vi "运维调试_总磷总氮.vi"() -> ()   [LabVIEW 2016, in "斯坦道总磷.lvlib"]
uses:
  <vilib>/Utility/miscctls.llb/LVStringsAndValuesArrayTypeDef_U16.ctl
  <vilib>/Utility/miscctls.llb/LVPointTypeDef.ctl
  <vilib>/Plasmionique/MB Master/MB_Master/MB_Master.lvclass
  <vilib>/Utility/config.llb/NI_LVConfig.lvlib
  <vilib>/ptbypt/NI_PtbyPt.lvlib
panel:
  in  "灯值调整":bool
  in  "测试量程配置":T1
  in  "启动参数设置":bool
  out "固件版本号":string
  in  "定时设置":cluster{"启动":bool, "控制命令":T2, "测量参数":T3}(xcontrol)
  out "模块版本号":string
  out "温度2":sgl
  out "温度1":sgl
  out "ADC":sgl
  out "F3":sgl format="%#.6f"
  out "F2":sgl format="%#.6f"
  out "F1":sgl format="%#.6f"
  out "F0":sgl format="%#.6f"
  out "运行状态":T4 {"数据时间:" format="%<%y/%m/%d %H:%M:%S>T"; "仪器时间:" format="%<%y/%m/%d %H:%M:%S>T"}
  in  "单选按钮":enum32{"COD", "NH3N", "TN", "TP"}(radio)=enum."TN"
  in  "仪器参数":bool
  out "二级权限":bool
  out "一级权限":bool
  out "输入密码":u32
  out "布尔":bool
  in  "流程固件":bool
  in  "量程参数读取":T5
  in  "模块启用":bool
  in  "串口设置":bool
  in  "公式一键写入":bool
  in  "流程路径":path=path "data/流程.xml"
  in  "曲线模型":cluster{"X^2":dbl, "X":dbl, "B":dbl, "r^2":dbl}(xcontrol)
  out "字符串 2":string
  in  "质控参数设置":bool
  in  "数组":string[](array[string])
  in  "量程切换阈值写入":bool
  in  "量程切换阈值读取":bool
  in  "参数下拉列表":enum16{"COD", "氨氮", "总氮", "总磷"}(ring)
  in  "量程下拉列表":enum16{"低量程", "高量程"}(ring)
  in  "测量模式下拉列表":enum16{"水样测量", "零点核查", "跨度核查", "标样核查", "加标回收"}(ring)
  in  "公式":cluster{"X^2":dbl, "X":dbl, "b":dbl}
  in  "写公式":bool
  in  "读公式":bool
  in  "返回":bool
  in  "参数设置":bool
  out "集成报警信息":string
  in  "停止":bool
  in  "手动启动":bool
  in  "单步测试":bool
  out "多列列表框":i32(listbox)
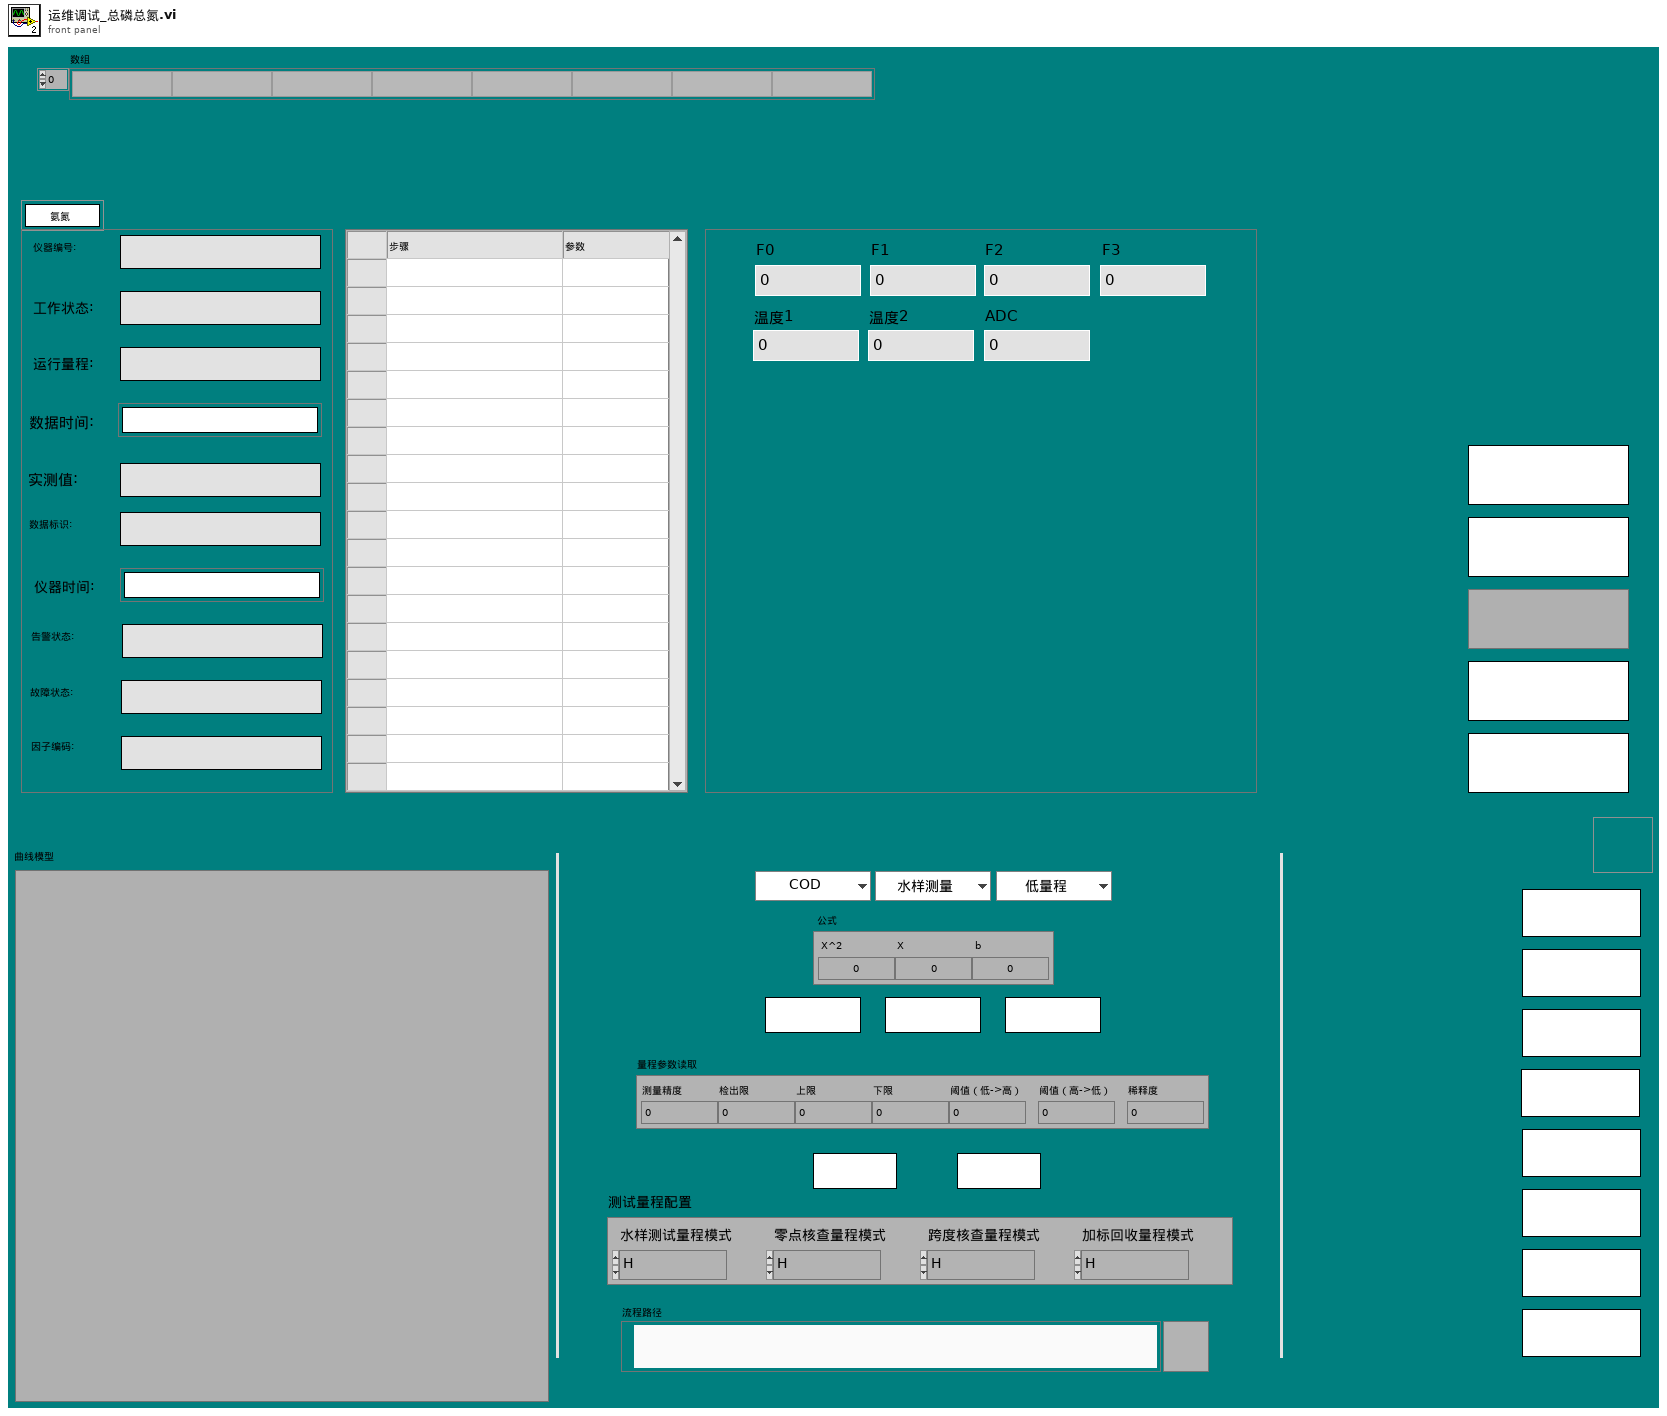
[diagram p1: front panel]
types:
  T1 = cluster{"水样测试量程模式":enum16{"H", "L", "AUTO"}, "空白核查量程模式":enum16{"H", "L", "AUTO"}, "跨度核查量程模式":enum16{"H", "L", "AUTO"}, "跨度核查量程模式 2":enum16{"H", "L", "AUTO"}}
  T2 = typedef "定时设置.xctl/国标控制命令.ctl" = enum16{"启动测量", "标样核查", "零点核查", "跨度核查", "空白测试", "平行样测试", "加标回收", "空白校准", "标样校准", "初始化（清洗）", "停止测试", "仪器重启", "校时", "模式设置", "测量间隔设置"}
  T3 = typedef "定时设置.xctl/测量参数.ctl" = u16
  T4 = cluster{"仪器编号:":string, "工作状态:":string, "运行量程: ":string, "数据时间:":timestamp, "实测值:":string, "数据标识: ":string, "仪器时间:":timestamp, "告警状态: ":string, "故障状态:  ":string, "因子编码:":string}
  T5 = cluster{"测量精度":dbl, "检出限":dbl, "上限":dbl, "下限":dbl, "阈值（低->高）":dbl, "阈值（高->低）":dbl, "稀释度":dbl}
  T6 = cluster{"时间源选择":enum16{"系统时间源", "仪器时间源"}, "外部时间源":timestamp}
  T7 = cluster{"系统时间":timestamp, "工作状态":enum16{"空闲", "水样测试", "标样核查", "零点核查", "跨度核查", "空白测试", "平行样测试", "加标回收", "空白校准", "标样校准", "初始化（清洗）"}, "测量模式":enum16{"待机", "连续模式", "周期模式", "定点模式", "受控模式", "手动模式"}, "告警代码":u16, "故障代码":u16, "日志代码":u16, "软件版本":u16, "F0":sgl, "F1":sgl, "F2":sgl, "F3":sgl, "T":sgl, "H":sgl, "id":u16, "flowid":u16, "量程":u16, "总磷控温温度1":sgl, "营养盐控温温度2":sgl, "ADC":sgl}
  T8 = enum32{"Bad", "Idle", "Run top level", "Running"}
  T9 = enum16{"空闲", "水样测试", "标样核查", "零点核查", "跨度核查", "空白测试", "平行样测试", "加标回收", "空白校准", "标样校准", "初始化（清洗）"}
  T10 = cluster{"水样测试量程模式":enum16{"H", "L", "AUTO"}, "空白核查量程模式":enum16{"H", "L", "AUTO"}, "跨度核查量程模式":enum16{"H", "L", "AUTO"}, "加标回收量程模式":enum16{"H", "L", "AUTO"}}
  T11 = typedef "LVStringsAndValuesArrayTypeDef_U16.ctl" = cluster{"String":string, "Value":u16}[]
  T12 = cluster{"COD":bool, "氨氮":bool, "总氮":bool, "总磷":bool}
  T13 = cluster{"参数下拉列表":enum16{"COD", "氨氮", "总氮", "总磷"}, "测量模式下拉列表":enum16{"水样测量", "零点核查", "跨度核查", "标样核查", "加标回收"}, "量程下拉列表":enum16{"低量程", "高量程"}}
  T14 = typedef "NI_LVConfig.lvlib/Config Data RefNum.ctl" = refnum<k1>
  T15 = cluster{"Major":u16, "Minor":u16, "Fix":u16, "Build":u16}
  T16 = typedef "LVPointTypeDef.ctl" = cluster{"Horizontal":i16, "Vertical":i16}
  T17 = cluster{"因子编码":u32, "单位":u16, "标样参考值":sgl, "水样数据时间":timestamp, "水样实测值":sgl, "水样数据标识":string, "标样数据时间":timestamp, "标样实测值":sgl, "标样数据标识":string, "空白数据时间":timestamp, "空白实测值":sgl, "空白数据标识":string, "零点核查数据时间":timestamp, "零点核查实测值":sgl, "零点核查数据标识":string, "跨度核查数据时间":timestamp, "跨度核查实测值":sgl, "跨度核查数据标识":string, "加标回收数据时间":timestamp, "加标回收实测值":sgl, "加标回收数据标识":string, "平行样数据时间":timestamp, "平行样实测值":sgl, "平行样数据标识":string, "F0":sgl, "F1":sgl, "F2":sgl, "F3":sgl, "F4":sgl, "F5":sgl, "F6":sgl, "F7":sgl, "温度":sgl, "湿度":sgl, "X值":sgl, "fidrange":u16}
  T18 = cluster{"时间标识":timestamp, "设备":string, "日志信息":string, "备注":string}
  T19 = cluster{"参数":string, "报警内容":string, "报警分析":string}
  T20 = cluster{"启动模式":enum16{"跨度核查", "水样测量", "空白核查", "标样核查", "加标回收"}, "启动参数":u16, "量程":enum16{"低量程", "高量程"}}
  T21 = cluster{"时间标识":timestamp, "设备":string, "日志信息":string, "流程参数":string}
  T22 = typedef "LVRowAndColumnUnsignedTypeDef.ctl" = cluster{"Row":u32, "Column":u32}
  T23 = cluster{"站号":u16, "量程切换":enum32{"H", "L", "AUTO"}, "控制命令":enum16{"启动测量", "标样核查", "零点核查", "跨度核查", "空白测试", "平行样测试", "加标回收", "空白校准", "标样校准", "初始化（清洗）", "停止测试", "仪器重启", "校时", "模式设置", "测量间隔设置"}, "模式设置":enum16{"待机", "连续模式", "周期模式", "定点模式", "受控模式", "手动模式"}, "测量间隔":u16}
  T24 = cluster{"被复制模型":cluster{"参数":u8, "测量模式":u8, "量程":u8}, "被覆盖模型":cluster{"参数":u8, "测量模式":u8, "量程":u8}[]}
  T25 = cluster{"总磷跨度值":dbl, "总磷零点标准液浓度":dbl, "总磷跨度标准液浓度":dbl, "总磷标准液标准浓度":dbl, "总氮跨度值":dbl, "总氮零点标准液浓度":dbl, "总氮跨度标准液浓度":dbl, "总氮标准液标准浓度":dbl, "COD跨度值":dbl, "COD零点标准液浓度":dbl, "COD跨度标准液浓度":dbl, "COD标准液标准浓度":dbl, "氨氮跨度值":dbl, "氨氮零点标准液浓度":dbl, "氨氮跨度标准液浓度":dbl, "氨氮标准液标准浓度":dbl}
  T26 = cluster{"测量量程":dbl, "测量精度":dbl, "测量间隔":dbl, "消解温度":dbl, "消解时长":dbl, "空白校准时间":timestamp, "曲线截距":dbl, "曲线斜率":dbl, "测量检出限":dbl, "测量信号值":dbl, "线性相关系数":dbl, "二次多项式系数":dbl, "标样校准时间":timestamp, "稀释倍数":dbl, "三项式系数":dbl, "空白标定系数":dbl, "量程系数":dbl, "F0/ORPA":dbl, "F1/ORPB":dbl, "F2/ORPK":dbl, "F3":dbl, "F4":dbl, "F5":dbl, "F6":dbl, "F7":dbl, "X0/滴定数":dbl, "量程":dbl}
  T27 = cluster{"COD仪器参数":cluster{"测量量程":dbl, "测量精度":dbl, "测量间隔":dbl, "消解温度":dbl, "消解时长":dbl, "空白校准时间":timestamp, "曲线截距":dbl, "曲线斜率":dbl, "测量检出限":dbl, "测量信号值":dbl, "线性相关系数":dbl, "二次多项式系数":dbl, "标样校准时间":timestamp, "稀释倍数":dbl, "三项式系数":dbl, "空白标定系数":dbl, "量程系数":dbl, "F0/ORPA":dbl, "F1/ORPB":dbl, "F2/ORPK":dbl, "F3":dbl, "F4":dbl, "F5":dbl, "F6":dbl, "F7":dbl, "X0/滴定数":dbl, "量程":dbl}, "氨氮仪器参数":cluster{"测量量程":dbl, "测量精度":dbl, "测量间隔":dbl, "消解温度":dbl, "消解时长":dbl, "空白校准时间":timestamp, "曲线截距":dbl, "曲线斜率":dbl, "测量检出限":dbl, "测量信号值":dbl, "线性相关系数":dbl, "二次多项式系数":dbl, "标样校准时间":timestamp, "稀释倍数":dbl, "三项式系数":dbl, "空白标定系数":dbl, "量程系数":dbl, "F0/ORPA":dbl, "F1/ORPB":dbl, "F2/ORPK":dbl, "F3":dbl, "F4":dbl, "F5":dbl, "F6":dbl, "F7":dbl, "X0/滴定数":dbl, "量程":dbl}, "总氮仪器参数":cluster{"测量量程":dbl, "测量精度":dbl, "测量间隔":dbl, "消解温度":dbl, "消解时长":dbl, "空白校准时间":timestamp, "曲线截距":dbl, "曲线斜率":dbl, "测量检出限":dbl, "测量信号值":dbl, "线性相关系数":dbl, "二次多项式系数":dbl, "标样校准时间":timestamp, "稀释倍数":dbl, "三项式系数":dbl, "空白标定系数":dbl, "量程系数":dbl, "F0/ORPA":dbl, "F1/ORPB":dbl, "F2/ORPK":dbl, "F3":dbl, "F4":dbl, "F5":dbl, "F6":dbl, "F7":dbl, "X0/滴定数":dbl, "量程":dbl}, "总磷仪器参数":cluster{"测量量程":dbl, "测量精度":dbl, "测量间隔":dbl, "消解温度":dbl, "消解时长":dbl, "空白校准时间":timestamp, "曲线截距":dbl, "曲线斜率":dbl, "测量检出限":dbl, "测量信号值":dbl, "线性相关系数":dbl, "二次多项式系数":dbl, "标样校准时间":timestamp, "稀释倍数":dbl, "三项式系数":dbl, "空白标定系数":dbl, "量程系数":dbl, "F0/ORPA":dbl, "F1/ORPB":dbl, "F2/ORPK":dbl, "F3":dbl, "F4":dbl, "F5":dbl, "F6":dbl, "F7":dbl, "X0/滴定数":dbl, "量程":dbl}}
  T28 = cluster{"测量精度":u16, "检出限":dbl, "上限":dbl, "下限":dbl, "阈值（低->高）":dbl, "阈值（高->低）":dbl, "稀释度":dbl}
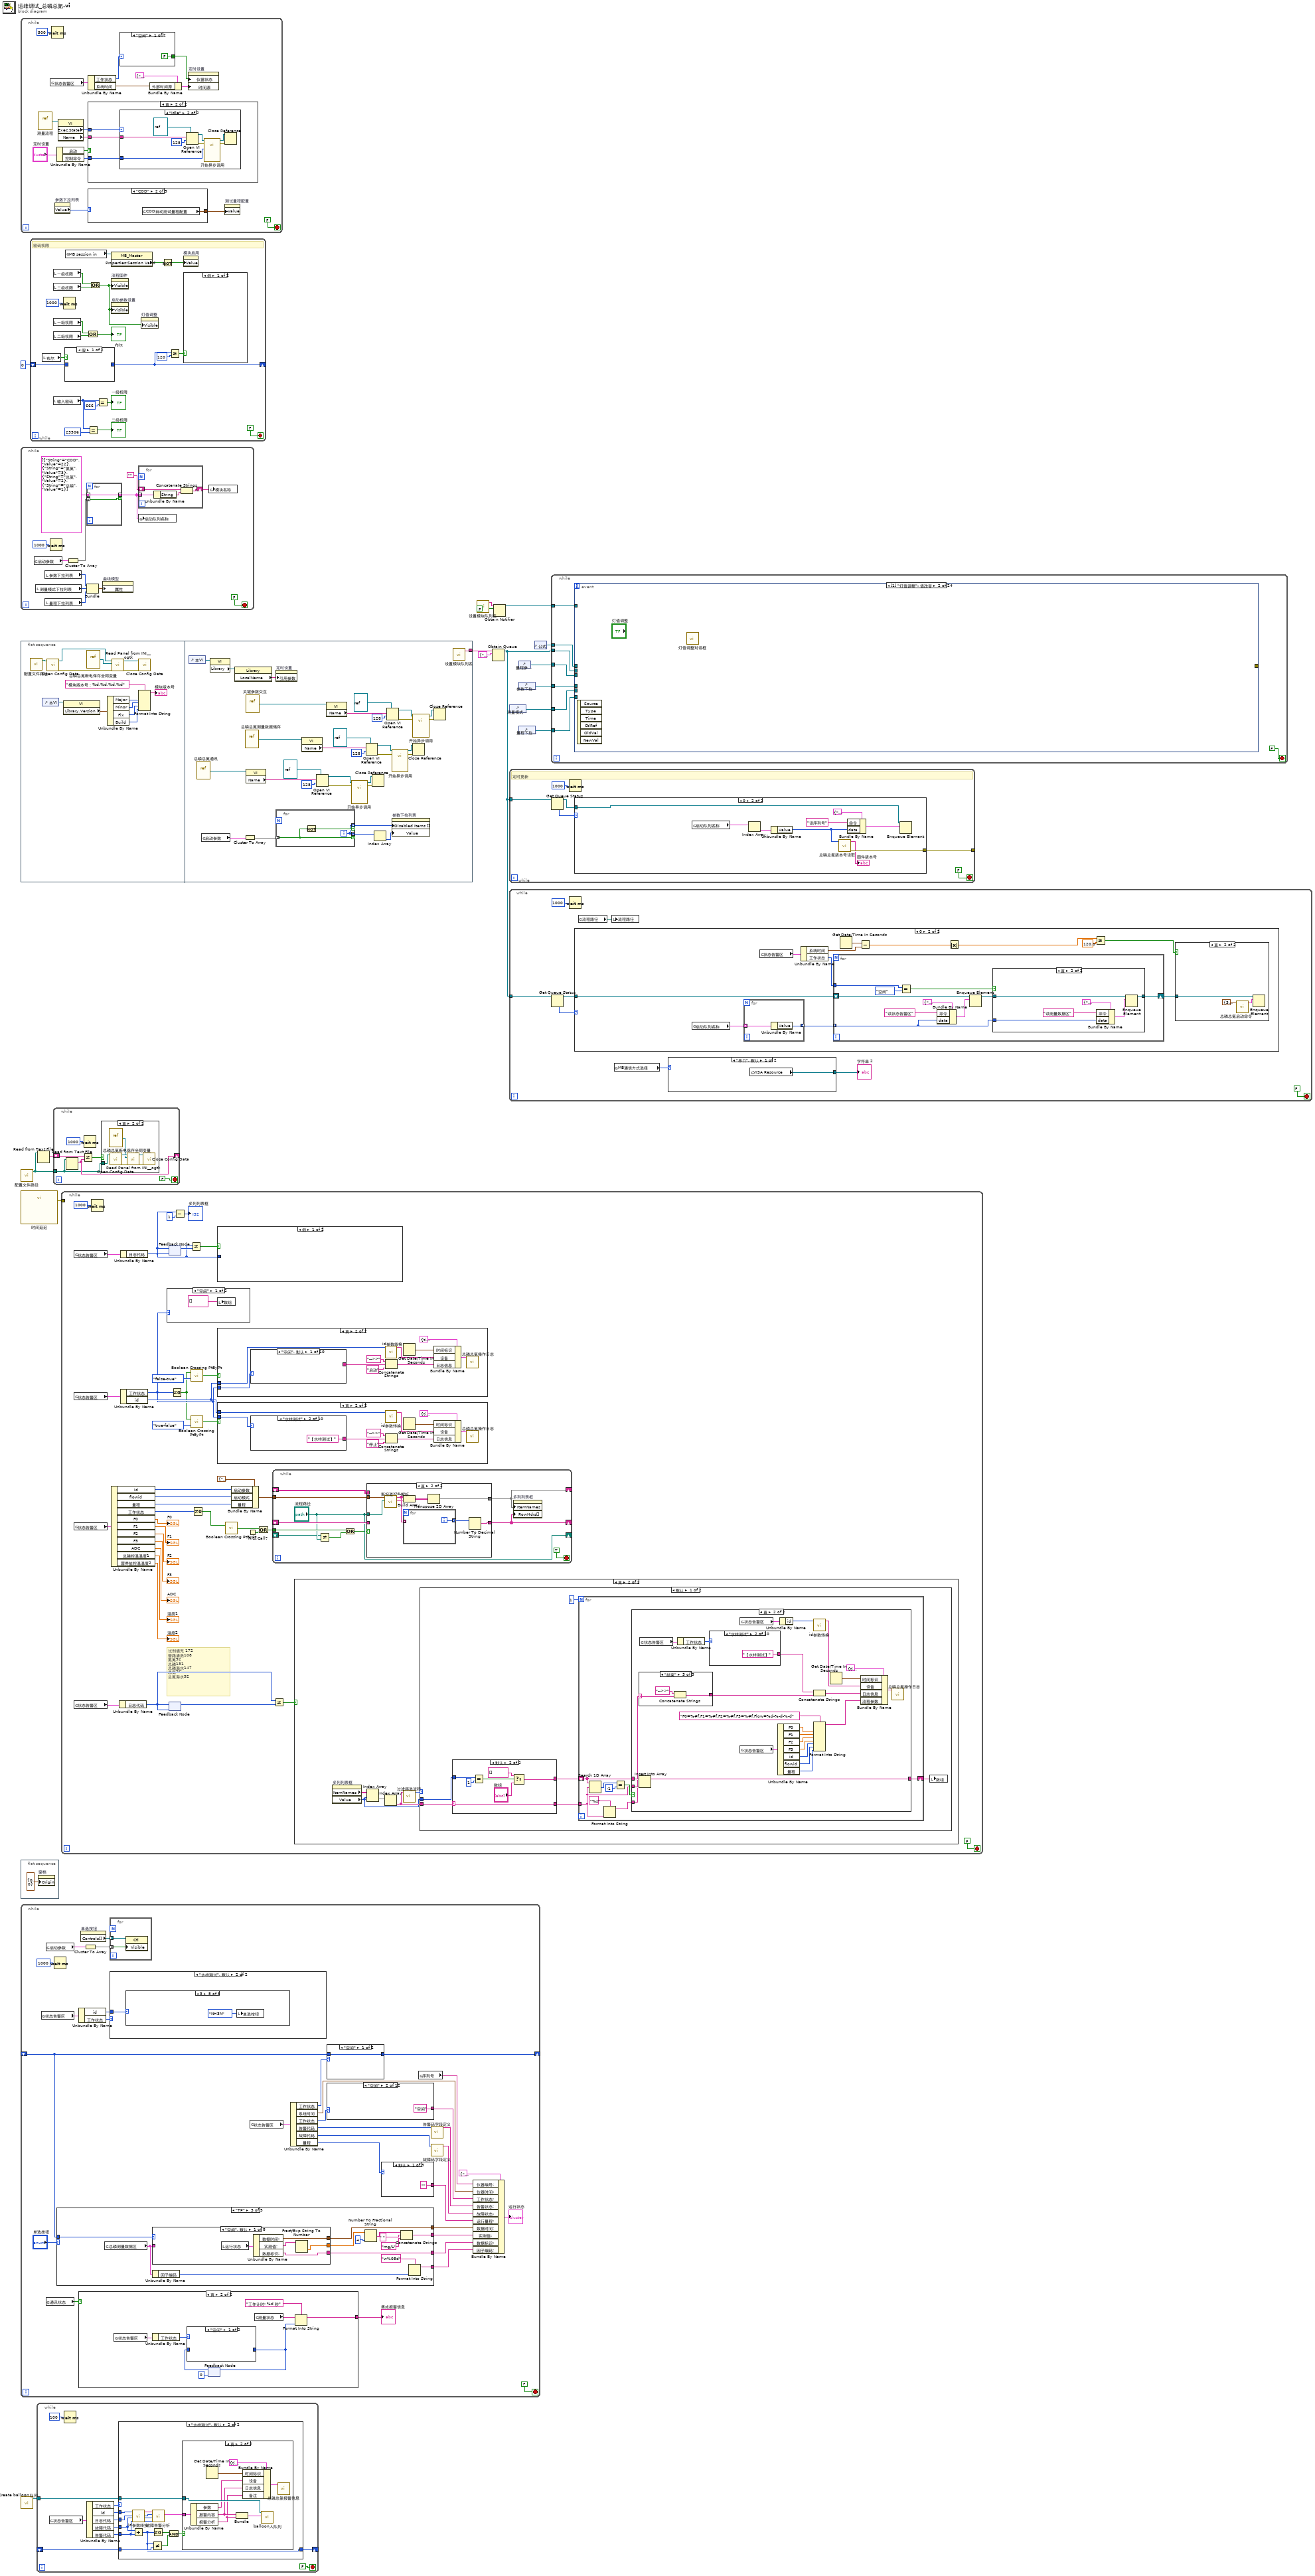
[diagram p0: block diagram]
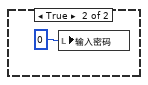
[diagram p5: hidden frame]
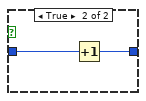
[diagram p6: hidden frame]
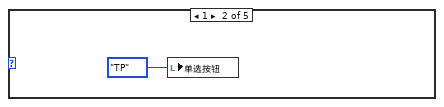
[diagram p11: hidden frame]
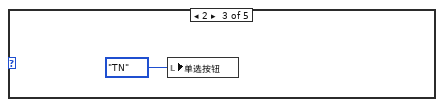
[diagram p12: hidden frame]
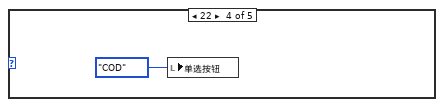
[diagram p13: hidden frame]
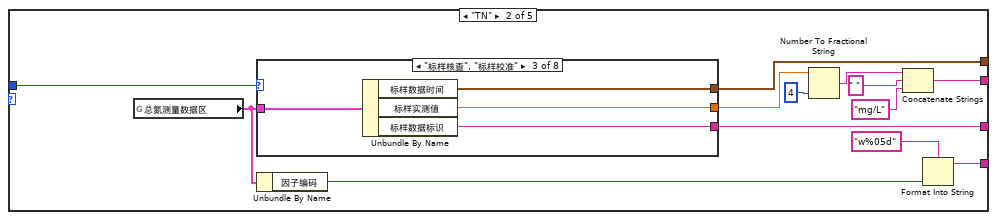
[diagram p15: hidden frame]
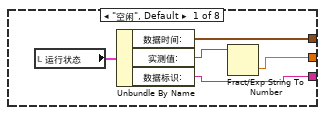
[diagram p16: hidden frame]
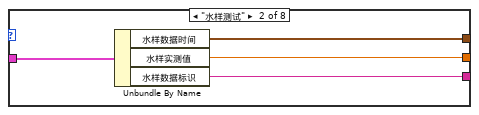
[diagram p17: hidden frame]
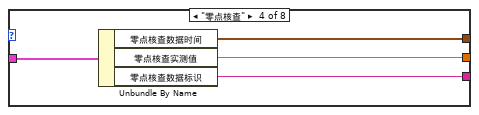
[diagram p18: hidden frame]
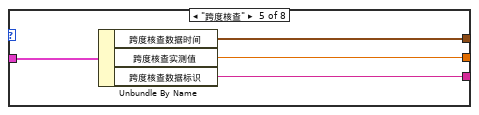
[diagram p19: hidden frame]
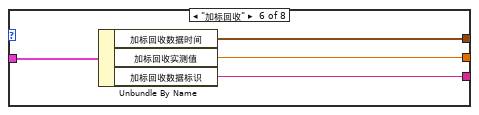
[diagram p20: hidden frame]
diagram:
  n1 = while {
    stop <- FALSE stop-if-true
    n2 = vi-ref "测量流程.vi"() -> (w30:refnum<vi>)
    n3 = global read "VAR总磷总氮全局变量.vi" "状态告警区"() -> (w27:T7)
    n4 = Wait (ms)(milliseconds to wait=u32 500 ("等待时间（毫秒）")) -> ()  [unwired: 1 out]
    n5 = property on="参数下拉列表" class="Enum (严格)"() -> ("Value"=w19:enum16{"COD", "氨氮", "总氮", "总磷"})  [unwired: 2 in, 2 out]
    n6 = Unbundle By Name("定时设置") -> ("启动"=w24:bool, "控制命令"=w23:T2)
    n7 = property class="VI"(reference=w30) -> ("Exec.State"=w29:T8, "Name"=w28:string)  [unwired: 1 in, 2 out]
    n8 = Unbundle By Name(w27) -> ("工作状态"=w26:T9, "系统时间"=w21:timestamp)
    n9 = case shown="真" w24 {
      tunnel: w28 -> [_ w41]
      tunnel: w23 -> [_ w40]
      tunnel: w29 -> [_ w39]
      frame False {
      }
      frame True {
        n10 = case shown="\"Idle\"" w39 {
          tunnel: w41 -> [_ w45]
          tunnel: w40 -> [_ w42]
          frame "Bad", Default {
          }
          frame "Idle" {
            n11 = Open VI Reference(type specifier VI Refnum (for type only)=refnum<vi> refnum, vi path=w45, options=128 ("选项")) -> (vi reference=w46:refnum<vi>, error out=w47:errorcluster)  [unwired: 3 in]
            n12 = call-by-ref "开始异步调用"(reference=w46, error in=w47, "控制命令"=w42) -> (reference out=w48:refnum<vi>, error out=w49:errorcluster)  [unwired: 11 in]
            n13 = Close Reference(reference=w48, error in (no error)=w49) -> ()  [unwired: 1 out]
          }
        }
      }
    }
    n14 = case shown="\"COD\"" w19 {
      tunnel: [_ w33 w34 w35 w36] -> w18
      frame Default {
      }
      frame "COD" {
        n15 = global read "总磷总氮断电保存全局变量.vi" "COD自动测试量程配置"() -> (w33:T10)
      }
      frame "氨氮" {
        n16 = global read "总磷总氮断电保存全局变量.vi" "氨氮自动测试量程配置"() -> (w34:T10)
      }
      frame "总氮" {
        n17 = global read "总磷总氮断电保存全局变量.vi" "总氮自动测试量程配置"() -> (w35:T10)
      }
      frame "总磷" {
        n18 = global read "总磷总氮断电保存全局变量.vi" "总磷自动测试量程配置"() -> (w36:T10)
      }
    }
    n19 = case shown="\"空闲\"" w26 {
      tunnel: [FALSE TRUE] -> w17
      frame "空闲" {
      }
      frame "水样测试", Default {
      }
    }
    n20 = Bundle By Name(cluster=T6 {"时间源选择"=enum."仪器时间源", "外部时间源"=timestamp(0 s since 1904-01-01)} ("时间源"), "外部时间源"=w21) -> (w20:T6)
    n21 = property on="定时设置" class="定时设置 (严格)"("仪器状态"=w17, "时间源"=w20) -> ()  [unwired: 2 in, 2 out]
    n22 = property on="测试量程配置" class="Clust (严格)"("Value"=w18) -> ()  [unwired: 2 in, 2 out]
  }
  n23 = while {
    stop <- FALSE stop-if-true
    n24 = global read "总磷总氮断电保存全局变量.vi" "启动参数"() -> (w59:T12)
    n25 = local read "测量模式下拉列表"() -> (w52:enum16{"水样测量", "零点核查", "跨度核查", "标样核查", "加标回收"})
    n26 = local read "参数下拉列表"() -> (w50:enum16{"COD", "氨氮", "总氮", "总磷"})
    n27 = local read "量程下拉列表"() -> (w51:enum16{"低量程", "高量程"})
    n28 = Wait (ms)(milliseconds to wait=u32 1000 ("等待时间（毫秒）")) -> ()  [unwired: 1 out]
    n29 = Cluster To Array(cluster=w59) -> (array=w58:bool[])
    n30 = for {
      tunnel: w58 -> [w67] mode=indexing
      tunnel: T11 [{"String"="COD", "Value"=22}, {"String"="氨氮", "Value"=3}, {"String"="总氮", "Value"=2}, {"String"="总磷", "Value"=1}] ("字符串与值[]") -> [w66] mode=indexing
      tunnel: [w66] -> w56 mode=indexing if=w67
    }
    n31 = Bundle("参数下拉列表"=w50, "测量模式下拉列表"=w52, "量程下拉列表"=w51) -> (w53:T13)  [unwired: 1 in]
    n32 = property on="曲线模型" class="曲线模型 (严格)"("属性"=w53) -> ()  [unwired: 2 in, 2 out]
    n33 = for {
      tunnel: w56 -> [w65] mode=indexing
      shift-right: [w64] -> w54
      shift-left: "" -> [w62]
      n34 = Unbundle By Name(w65) -> ("String"=w63:string)
      n35 = Concatenate Strings(w62, w63) -> (w64:string)
    }
    n36 = global write "VAR总磷总氮全局变量.vi" "启动队列名称"(w56) -> ()
    n37 = global write "VAR总磷总氮全局变量.vi" "模块名称"(w54) -> ()
  }
  n38 = flat-sequence {
    tunnel: [w83] -> w6
    frame #0 {
      n39 = call "配置文件路径.vi"() -> ("appended path"=w76:path)  [unwired: 11 in]
      n40 = control-ref of="本VI"() -> (w75:refnum<vi>)
      n41 = call <vilib>:"Open Config Data.vi"("configuration file path"=w76) -> ("error out"=w80:errorcluster, "refnum"=w77:T14)  [unwired: 8 in, 1 out]
      n42 = property class="VI"(reference=w75) -> ("Library.Version"=w74:T15)  [unwired: 1 in, 2 out]
      n43 = vi-ref "总磷总氮断电保存全局变量.vi"() -> (w78:refnum<vi>)
      n44 = Unbundle By Name(w74) -> ("Major"=w72:u16, "Minor"=w71:u16, "Fix"=w70:u16, "Build"=w69:u16)
      n45 = call <userlib>:"Read Panel from INI__ogtk.vi"("error in (no error)"=w80, "VI ref"=w78, "refnum"=w77) -> ("error out"=w81:errorcluster, "refnum out"=w79:T14)  [unwired: 7 in]
      n46 = call <vilib>:"Close Config Data.vi"("error in (no error)"=w81, "refnum"=w79) -> ()  [unwired: 8 in, 2 out]
      n47 = Format Into String(format string="模块版本号：%d.%d.%d.%d" ("格式字符串"), w72, w71, w70, w69) -> (resulting string=→"模块版本号":string)  [unwired: 2 in, 1 out]
    }
    frame #1 {
      n48 = control-ref of="本VI"() -> (w84:refnum<vi>)
      n49 = vi-ref "总磷总氮通讯.vi"() -> (w99:refnum<vi>)
      n50 = global read "总磷总氮断电保存全局变量.vi" "启动参数"() -> (w87:T12)
      n51 = property class="VI"(reference=w84) -> ("Library"=w85:refnum<vi>)  [unwired: 1 in, 2 out]
      n52 = property class="Library"(reference=w85) -> ("LocalName"=w86:string)  [unwired: 1 in, 2 out]
      n53 = Cluster To Array(cluster=w87) -> (array=w88:bool[])
      n54 = vi-ref "总磷总氮测量数据储存.vi"() -> (w107:refnum<vi>)
      n55 = vi-ref "关键参数交互.vi"() -> (w98:refnum<vi>)
      n56 = property class="VI"(reference=w99) -> ("Name"=w100:string)  [unwired: 1 in, 2 out]
      n57 = property on="定时设置" class="定时设置 (严格)"("引用参数"=w86) -> ()  [unwired: 2 in, 2 out]
      n58 = for {
        tunnel: w88 -> [w115] mode=indexing
        tunnel: [w116] -> w90 mode=indexing if=w117
        tunnel: [w116] -> w89 mode=indexing if=w115
        i -> [w116]
        n59 = Not(x=w115) -> (.not. x?=w117:bool)
      }
      n60 = property class="VI"(reference=w107) -> ("Name"=w114:string)  [unwired: 1 in, 2 out]
      n61 = Open VI Reference(type specifier VI Refnum (for type only)=refnum<vi> refnum, vi path=w100, options=128 ("选项")) -> (vi reference=w102:refnum<vi>, error out=w104:errorcluster)  [unwired: 3 in]
      n62 = property class="VI"(reference=w98) -> ("Name"=w92:string)  [unwired: 1 in, 2 out]
      n63 = call-by-ref "开始异步调用"(reference=w102, error in=w104) -> (reference out=w106:refnum<vi>, error out=w105:errorcluster)  [unwired: 12 in]
      n64 = Open VI Reference(type specifier VI Refnum (for type only)=refnum<vi> refnum, vi path=w114, options=128 ("选项")) -> (vi reference=w112:refnum<vi>, error out=w110:errorcluster)  [unwired: 3 in]
      n65 = Close Reference(reference=w106, error in (no error)=w105) -> ()  [unwired: 1 out]
      n66 = Index Array(array=w89) -> (element=w82:i32)  [unwired: 1 in]
      n67 = Open VI Reference(type specifier VI Refnum (for type only)=refnum<vi> refnum, vi path=w92, options=128 ("选项")) -> (vi reference=w94:refnum<vi>, error out=w95:errorcluster)  [unwired: 3 in]
      n68 = call-by-ref "开始异步调用"(reference=w112, error in=w110) -> (reference out=w108:refnum<vi>, error out=w109:errorcluster)  [unwired: 12 in]
      n69 = property on="参数下拉列表" class="Enum (严格)"("Disabled Items []"=w90, "Value"=w82) -> ()  [unwired: 2 in, 2 out]
      n70 = call-by-ref "开始异步调用"(reference=w94, error in=w95) -> (reference out=w97:refnum<vi>, error out=w96:errorcluster)  [unwired: 12 in]
      n71 = Close Reference(reference=w108, error in (no error)=w109) -> ()  [unwired: 1 out]
      n72 = Close Reference(reference=w97, error in (no error)=w96) -> ()  [unwired: 1 out]
      n73 = call "设置模块队列名.vi"() -> ("Msg"=w83:string)  [unwired: 5 in]
    }
  }
  n74 = call "配置文件路径.vi"() -> ("appended path"=w4:path)  [unwired: 11 in]
  n75 = call "时间延迟"() -> ("error out"=w11:errorcluster)  [unwired: 11 in]
  n76 = flat-sequence {
    frame #0 {
      n77 = property on="窗格" class="Pane"("Origin"=T16 {"Horizontal"=0, "Vertical"=0} ("原点")) -> ()  [unwired: 2 in, 2 out]
    }
  }
  n78 = while {
    shift-right: [w120] -> _
    shift-left: _ -> [w119]
    stop <- FALSE stop-if-true
    n79 = global read "VAR总磷总氮全局变量.vi" "状态告警区"() -> (w131:T7)
    n80 = global read "总磷总氮断电保存全局变量.vi" "启动参数"() -> (w123:T12)
    n81 = global read "VAR总磷总氮全局变量.vi" "通讯状态"() -> (w147:bool)
    n82 = Wait (ms)(milliseconds to wait=u32 1000 ("等待时间（毫秒）")) -> ()  [unwired: 1 out]
    n83 = case shown="\"TP\"" "单选按钮" {
      tunnel: w119 -> [_ w163 w209 w255 w301]
      tunnel: [_ w162 w208 w253 w299] -> w135
      tunnel: [_ w161 w211 w257 w303] -> w134
      tunnel: [_ w160 w206 w251 w297] -> w133
      tunnel: [_ w159 w210 w256 w302] -> w132
      frame Default {
      }
      frame "TN" {
        n84 = global read "VAR总磷总氮全局变量.vi" "总氮测量数据区"() -> (w164:T17)
        n85 = case shown="\"标样核查\", \"标样校准\"" w163 {
          tunnel: [w174 w180 w184 w188 w192 w196 w200 w204] -> w162
          tunnel: [w172 w179 w183 w187 w190 w195 w199 w203] -> w166
          tunnel: [w175 w178 w182 w186 w189 w194 w198 w202] -> w160
          tunnel: w164 -> [_ w177 w181 w185 w191 w193 w197 w201]
          frame "空闲", Default {
            n86 = local read "运行状态"() -> (w176:T4)
            n87 = Unbundle By Name(w176) -> ("数据时间:"=w174:timestamp, "实测值:"=w173:string, "数据标识:"=w175:string)
            n88 = Fract/Exp String To Number(string=w173) -> (number=w172:dbl)  [unwired: 3 in, 1 out]
          }
          frame "水样测试" {
            n89 = Unbundle By Name(w177) -> ("水样数据时间"=w180:timestamp, "水样实测值"=w179:sgl, "水样数据标识"=w178:string)
          }
          frame "标样核查", "标样校准" {
            n90 = Unbundle By Name(w181) -> ("标样数据时间"=w184:timestamp, "标样实测值"=w183:sgl, "标样数据标识"=w182:string)
          }
          frame "零点核查" {
            n91 = Unbundle By Name(w185) -> ("零点核查数据时间"=w188:timestamp, "零点核查实测值"=w187:sgl, "零点核查数据标识"=w186:string)
          }
          frame "跨度核查" {
            n92 = Unbundle By Name(w191) -> ("跨度核查数据时间"=w192:timestamp, "跨度核查实测值"=w190:sgl, "跨度核查数据标识"=w189:string)
          }
          frame "加标回收" {
            n93 = Unbundle By Name(w193) -> ("加标回收数据时间"=w196:timestamp, "加标回收实测值"=w195:sgl, "加标回收数据标识"=w194:string)
          }
          frame "空白测试", "空白校准" {
            n94 = Unbundle By Name(w197) -> ("空白数据时间"=w200:timestamp, "空白实测值"=w199:sgl, "空白数据标识"=w198:string)
          }
          frame "平行样测试" {
            n95 = Unbundle By Name(w201) -> ("平行样数据时间"=w204:timestamp, "平行样实测值"=w203:sgl, "平行样数据标识"=w202:string)
          }
        }
        n96 = Unbundle By Name(w164) -> ("因子编码"=w170:u32)
        n97 = Number To Fractional String(number=w166, precision (6)=i16 4 ("精度(6)")) -> (F-format string=w168:string)  [unwired: 2 in]
        n98 = Concatenate Strings(w168, " " ("字符串"), "mg/L" ("字符串")) -> (w161:string)
        n99 = Format Into String(format string="w%05d" ("格式字符串"), w170) -> (resulting string=w159:string)  [unwired: 2 in, 1 out]
      }
      frame "TP" {
        n100 = global read "VAR总磷总氮全局变量.vi" "总磷测量数据区"() -> (w205:T17)
        n101 = case shown="\"空闲\", 默认" w209 {
          tunnel: [w220 w226 w230 w234 w238 w242 w246 w250] -> w208
          tunnel: [w218 w225 w229 w233 w236 w241 w245 w249] -> w207
          tunnel: [w221 w224 w228 w232 w235 w240 w244 w248] -> w206
          tunnel: w205 -> [_ w223 w227 w231 w237 w239 w243 w247]
          frame "空闲", Default {
            n102 = local read "运行状态"() -> (w222:T4)
            n103 = Unbundle By Name(w222) -> ("数据时间:"=w220:timestamp, "实测值:"=w219:string, "数据标识:"=w221:string)
            n104 = Fract/Exp String To Number(string=w219) -> (number=w218:dbl)  [unwired: 3 in, 1 out]
          }
          frame "水样测试" {
            n105 = Unbundle By Name(w223) -> ("水样数据时间"=w226:timestamp, "水样实测值"=w225:sgl, "水样数据标识"=w224:string)
          }
          frame "标样核查" {
            n106 = Unbundle By Name(w227) -> ("标样数据时间"=w230:timestamp, "标样实测值"=w229:sgl, "标样数据标识"=w228:string)
          }
          frame "零点核查" {
            n107 = Unbundle By Name(w231) -> ("零点核查数据时间"=w234:timestamp, "零点核查实测值"=w233:sgl, "零点核查数据标识"=w232:string)
          }
          frame "跨度核查" {
            n108 = Unbundle By Name(w237) -> ("跨度核查数据时间"=w238:timestamp, "跨度核查实测值"=w236:sgl, "跨度核查数据标识"=w235:string)
          }
          frame "加标回收" {
            n109 = Unbundle By Name(w239) -> ("加标回收数据时间"=w242:timestamp, "加标回收实测值"=w241:sgl, "加标回收数据标识"=w240:string)
          }
          frame "空白测试" {
            n110 = Unbundle By Name(w243) -> ("空白数据时间"=w246:timestamp, "空白实测值"=w245:sgl, "空白数据标识"=w244:string)
          }
          frame "平行样测试" {
            n111 = Unbundle By Name(w247) -> ("平行样数据时间"=w250:timestamp, "平行样实测值"=w249:sgl, "平行样数据标识"=w248:string)
          }
        }
        n112 = Unbundle By Name(w205) -> ("因子编码"=w216:u32)
        n113 = Number To Fractional String(number=w207, precision (6)=i16 4 ("精度(6)")) -> (F-format string=w214:string)  [unwired: 2 in]
        n114 = Concatenate Strings(w214, " " ("字符串"), "mg/L" ("字符串")) -> (w211:string)
        n115 = Format Into String(format string="w%05d" ("格式字符串"), w216) -> (resulting string=w210:string)  [unwired: 2 in, 1 out]
      }
      frame "NH3N" {
        n116 = global read "VAR总磷总氮全局变量.vi" "氨氮测量数据区"() -> (w254:T17)
        n117 = case shown="\"空闲\", 默认" w255 {
          tunnel: [w266 w272 w276 w280 w284 w288 w292 w296] -> w253
          tunnel: [w264 w271 w275 w279 w282 w287 w291 w295] -> w252
          tunnel: [w267 w270 w274 w278 w281 w286 w290 w294] -> w251
          tunnel: w254 -> [_ w269 w273 w277 w283 w285 w289 w293]
          frame "空闲", Default {
            n118 = local read "运行状态"() -> (w268:T4)
            n119 = Unbundle By Name(w268) -> ("数据时间:"=w266:timestamp, "实测值:"=w265:string, "数据标识:"=w267:string)
            n120 = Fract/Exp String To Number(string=w265) -> (number=w264:dbl)  [unwired: 3 in, 1 out]
          }
          frame "水样测试" {
            n121 = Unbundle By Name(w269) -> ("水样数据时间"=w272:timestamp, "水样实测值"=w271:sgl, "水样数据标识"=w270:string)
          }
          frame "标样核查" {
            n122 = Unbundle By Name(w273) -> ("标样数据时间"=w276:timestamp, "标样实测值"=w275:sgl, "标样数据标识"=w274:string)
          }
          frame "零点核查" {
            n123 = Unbundle By Name(w277) -> ("零点核查数据时间"=w280:timestamp, "零点核查实测值"=w279:sgl, "零点核查数据标识"=w278:string)
          }
          frame "跨度核查" {
            n124 = Unbundle By Name(w283) -> ("跨度核查数据时间"=w284:timestamp, "跨度核查实测值"=w282:sgl, "跨度核查数据标识"=w281:string)
          }
          frame "加标回收" {
            n125 = Unbundle By Name(w285) -> ("加标回收数据时间"=w288:timestamp, "加标回收实测值"=w287:sgl, "加标回收数据标识"=w286:string)
          }
          frame "空白测试" {
            n126 = Unbundle By Name(w289) -> ("空白数据时间"=w292:timestamp, "空白实测值"=w291:sgl, "空白数据标识"=w290:string)
          }
          frame "平行样测试" {
            n127 = Unbundle By Name(w293) -> ("平行样数据时间"=w296:timestamp, "平行样实测值"=w295:sgl, "平行样数据标识"=w294:string)
          }
        }
        n128 = Unbundle By Name(w254) -> ("因子编码"=w262:u32)
        n129 = Number To Fractional String(number=w252, precision (6)=i16 4 ("精度(6)")) -> (F-format string=w260:string)  [unwired: 2 in]
        n130 = Concatenate Strings(w260, " " ("字符串"), "mg/L" ("字符串")) -> (w257:string)
        n131 = Format Into String(format string="w%05d" ("格式字符串"), w262) -> (resulting string=w256:string)  [unwired: 2 in, 1 out]
      }
      frame "COD" {
        n132 = global read "VAR总磷总氮全局变量.vi" "COD测量数据区"() -> (w300:T17)
        n133 = case shown="\"空闲\", 默认" w301 {
          tunnel: [w312 w318 w322 w326 w330 w334 w338 w342] -> w299
          tunnel: [w310 w317 w321 w325 w328 w333 w337 w341] -> w298
          tunnel: [w313 w316 w320 w324 w327 w332 w336 w340] -> w297
          tunnel: w300 -> [_ w315 w319 w323 w329 w331 w335 w339]
          frame "空闲", Default {
            n134 = local read "运行状态"() -> (w314:T4)
            n135 = Unbundle By Name(w314) -> ("数据时间:"=w312:timestamp, "实测值:"=w311:string, "数据标识:"=w313:string)
            n136 = Fract/Exp String To Number(string=w311) -> (number=w310:dbl)  [unwired: 3 in, 1 out]
          }
          frame "水样测试" {
            n137 = Unbundle By Name(w315) -> ("水样数据时间"=w318:timestamp, "水样实测值"=w317:sgl, "水样数据标识"=w316:string)
          }
          frame "标样核查" {
            n138 = Unbundle By Name(w319) -> ("标样数据时间"=w322:timestamp, "标样实测值"=w321:sgl, "标样数据标识"=w320:string)
          }
          frame "零点核查" {
            n139 = Unbundle By Name(w323) -> ("零点核查数据时间"=w326:timestamp, "零点核查实测值"=w325:sgl, "零点核查数据标识"=w324:string)
          }
          frame "跨度核查" {
            n140 = Unbundle By Name(w329) -> ("跨度核查数据时间"=w330:timestamp, "跨度核查实测值"=w328:sgl, "跨度核查数据标识"=w327:string)
          }
          frame "加标回收" {
            n141 = Unbundle By Name(w331) -> ("加标回收数据时间"=w334:timestamp, "加标回收实测值"=w333:sgl, "加标回收数据标识"=w332:string)
          }
          frame "空白测试" {
            n142 = Unbundle By Name(w335) -> ("空白数据时间"=w338:timestamp, "空白实测值"=w337:sgl, "空白数据标识"=w336:string)
          }
          frame "平行样测试" {
            n143 = Unbundle By Name(w339) -> ("平行样数据时间"=w342:timestamp, "平行样实测值"=w341:sgl, "平行样数据标识"=w340:string)
          }
        }
        n144 = Unbundle By Name(w300) -> ("因子编码"=w308:u32)
        n145 = Number To Fractional String(number=w298, precision (6)=i16 4 ("精度(6)")) -> (F-format string=w306:string)  [unwired: 2 in]
        n146 = Concatenate Strings(w306, " " ("字符串"), "mg/L" ("字符串")) -> (w303:string)
        n147 = Format Into String(format string="w%05d" ("格式字符串"), w308) -> (resulting string=w302:string)  [unwired: 2 in, 1 out]
      }
    }
    n148 = Unbundle By Name(w131) -> ("id"=w130:u16, "工作状态"=w125:T9)
    n149 = case shown="真" w147 {
      tunnel: ["通讯异常" ("集成报警信息") w363] -> w146
      frame False {
      }
      frame True {
        n150 = global read "VAR总磷总氮全局变量.vi" "状态告警区"() -> (w369:T7)
        n151 = Unbundle By Name(w369) -> ("工作状态"=w368:T9)
        n152 = feedback #1(0) -> (w366:i32)
        n153 = case shown="\"空闲\"" w368 {
          tunnel: w366 -> [_ w371]
          tunnel: [_ w370] -> w364
          frame "空闲" {
          }
          frame Default {
            n154 = Increment(x=w371) -> (x+1=w370:i32)
          }
        }
        n155 = feedback-in #1(w364) -> ()
        n156 = global read "VAR总磷总氮全局变量.vi" "测量状态"() -> (w362:string)
        n157 = Format Into String(format string="工作计时: %d 秒" ("格式字符串"), initial string=w362, w364) -> (resulting string=w363:string)  [unwired: 1 in, 1 out]
      }
    }
    "集成报警信息" <- w146
    n158 = property on="单选按钮" class="RadioBtnsControl (严格)"() -> ("Controls[]"=w124:refnum<vi>[])  [unwired: 2 in, 2 out]
    n159 = Cluster To Array(cluster=w123) -> (array=w122:bool[])
    n160 = for {
      tunnel: w124 -> [w153] mode=indexing
      tunnel: w122 -> [w152] mode=indexing
      n161 = property class="Ctl"(reference=w153, "Visible"=w152) -> ()  [unwired: 1 in, 2 out]
    }
    n162 = case shown="\"水样测试\", 默认" w125 {
      tunnel: w130 -> [_ w154]
      frame "空闲" {
      }
      frame "水样测试", Default {
        n163 = case shown="3" w154 {
          frame 0, Default {
          }
          frame 1 {
            n164 = local write "单选按钮"(enum32{"COD", "NH3N", "TN", "TP"}."TP" ("单选按钮")) -> ()
          }
          frame 2 {
            n165 = local write "单选按钮"(enum32{"COD", "NH3N", "TN", "TP"}."TN" ("单选按钮")) -> ()
          }
          frame 22 {
            n166 = local write "单选按钮"(enum32{"COD", "NH3N", "TN", "TP"}."COD" ("单选按钮")) -> ()
          }
          frame 3 {
            n167 = local write "单选按钮"(enum32{"COD", "NH3N", "TN", "TP"}."NH3N" ("单选按钮")) -> ()
          }
        }
      }
    }
    n168 = global read "VAR总磷总氮全局变量.vi" "状态告警区"() -> (w145:T7)
    n169 = Unbundle By Name(w145) -> ("工作状态"=w121:T9, "系统时间"=w141:timestamp, "工作状态"=w140:T9, "告警代码"=w129:u16, "故障代码"=w127:u16, "量程"=w138:u16)
    n170 = case shown="\"空闲\"" w121 {
      selector: w121 -> [_ w151]
      tunnel: [w150 w151] -> w120
      tunnel: w119 -> [w150 _]
      frame "空闲" {
      }
      frame "水样测试", Default {
      }
    }
    n171 = case shown="\"空闲\"" w140 {
      selector: w140 -> [w346 _ _ _ _ _ _ _ _ _ _ _]
      tunnel: [w347 "空闲" ("工作状态") "水样测量" ("工作状态") "标样核查" ("工作状态") "零点核查" ("工作状态") "跨度核查" ("工作状态") "空白测试" ("工作状态") "平行样测试" ("工作状态") "加标回收" ("工作状态") "空白校准" ("工作状态") "标样校准" ("工作状态") "初始化" ("工作状态")] -> w139
      frame Default {
        n172 = Format Into String(format string="%d" ("格式字符串"), initial string="未知" ("工作状态"), w346) -> (resulting string=w347:string)  [unwired: 1 in, 1 out]
      }
      frame "空闲" {
      }
      frame "水样测试" {
      }
      frame "标样核查" {
      }
      frame "零点核查" {
      }
      frame "跨度核查" {
      }
      frame "空白测试" {
      }
      frame "平行样测试" {
      }
      frame "加标回收" {
      }
      frame "空白校准" {
      }
      frame "标样校准" {
      }
      frame "初始化（清洗）" {
      }
    }
    n173 = case shown="默认" w138 {
      tunnel: ["" ("字符串") "低量程" ("字符串") "高量程" ("字符串")] -> w137
      frame Default {
      }
      frame 0 {
      }
      frame 1 {
      }
    }
    n174 = global read "VAR总磷总氮全局变量.vi" "序列号"() -> (w142:string)
    n175 = call "告警码字段定义.vi"("告警代码"=w129) -> ("字符串"=w128:string)  [unwired: 8 in, 2 out]
    n176 = call "故障码字段定义.vi"("故障代码"=w127) -> ("字符串"=w126:string)  [unwired: 10 in]
    n177 = Bundle By Name(cluster=T4 {"仪器编号:"="", "工作状态:"="", "运行量程: "="", "数据时间:"=timestamp(0 s since 1904-01-01), "实测值:"="", "数据标识: "="", "仪器时间:"=timestamp(0 s since 1904-01-01), "告警状态: "="", "故障状态:  "="", "因子编码:"=""} ("运行状态"), "仪器编号:"=w142, "仪器时间:"=w141, "工作状态:"=w139, "告警状态:"=w128, "故障状态:"=w126, "运行量程:"=w137, "数据时间:"=w135, "实测值:"=w134, "数据标识:"=w133, "因子编码:"=w132) -> (→"运行状态":T4)
  }
  n178 = call "Create balloon 队列.vi"() -> ("队列输出"=w8:refnum<queue>)  [unwired: 11 in]
  n179 = while {
    shift-right: [w380] -> _
    shift-left: u32 0 ("y") -> [w382]
    stop <- FALSE stop-if-true
    # "密码权限"
    n180 = local read "布尔"() -> (w383:bool)
    n181 = local read "一级权限"() -> (w376:bool)
    n182 = local read "二级权限"() -> (w377:bool)
    n183 = local read "一级权限"() -> (w385:bool)
    n184 = local read "二级权限"() -> (w386:bool)
    n185 = local read "输入密码"() -> (w389:u32)
    n186 = Wait (ms)(milliseconds to wait=u32 1000 ("等待时间（毫秒）")) -> ()  [unwired: 1 out]
    n187 = case shown="假" w383 {
      tunnel: w382 -> [_ w395]
      tunnel: [_ w394] -> w380
      frame False {
      }
      frame True {
        n188 = Increment(x=w395) -> (x+1=w394:u32)
      }
    }
    n189 = global read "VAR总磷总氮全局变量.vi" "MB session in"() -> (w375:refnum<class "MB_Master.lvclass">)
    n190 = Or(x=w385, y=w386) -> (x .or. y?=→"布尔":bool)
    n191 = Equal?(x=w389, y=u32 23506) -> (x = y?=→"二级权限":bool)
    n192 = Or(x=w376, y=w377) -> (x .or. y?=w372:bool)
    n193 = Equal?(x=w389, y=u32 666) -> (x = y?=→"一级权限":bool)
    n194 = property class="MB_Master"(reference=w375) -> ("Properties:Session Valid"=w374:bool)  [unwired: 1 in, 2 out]
    n195 = property on="流程固件" class="Bool"("Visible"=w372) -> ()  [unwired: 2 in, 2 out]
    n196 = property on="启动参数设置" class="Bool"("Visible"=w372) -> ()  [unwired: 2 in, 2 out]
    n197 = property on="灯值调整" class="Bool"("Visible"=w372) -> ()  [unwired: 2 in, 2 out]
    n198 = Not(x=w374) -> (.not. x?=w373:bool)
    n199 = Greater Or Equal?(x=w380, y=u32 120) -> (x >= y?=w378:bool)
    n200 = property on="模块启用" class="Bool (严格)"("Value"=w373) -> ()  [unwired: 2 in, 2 out]
    n201 = case shown="假" w378 {
      frame False {
      }
      frame True {
        n202 = local write "输入密码"(u32 0 ("输入密码")) -> ()
      }
    }
  }
  n203 = while {
    tunnel: w8 -> [w402]
    shift-right: [w398] -> _
    shift-left: _ -> [w399]
    stop <- FALSE stop-if-true
    n204 = global read "VAR总磷总氮全局变量.vi" "状态告警区"() -> (w396:T7)
    n205 = Wait (ms)(milliseconds to wait=u32 100) -> ()  [unwired: 1 out]
    n206 = Unbundle By Name(w396) -> ("工作状态"=w397:T9, "id"=w404:u16, "日志代码"=w403:u16, "故障代码"=w401:u16, "告警代码"=w400:u16)
    n207 = case shown="\"水样测试\", 默认" w397 {
      tunnel: w404 -> [_ w419]
      tunnel: w403 -> [_ w418]
      tunnel: w402 -> [_ w415]
      tunnel: w401 -> [_ w414]
      tunnel: w400 -> [_ w413]
      tunnel: w399 -> [w407 w412]
      tunnel: [w407 w411] -> w398
      frame "空闲" {
      }
      frame "水样测试", Default {
        n208 = call "id参数转换.vi"("id"=w419) -> ("table输出"=w416:string)  [unwired: 10 in]
        n209 = Add(x=w414, y=w413) -> (x+y=w411:u16)
        n210 = Not Equal?(x=w411, y=w412) -> (x != y?=w409:bool)
        n211 = Not Equal To 0?(x=w411) -> (x != 0?=w410:bool)
        n212 = call "故障告警分析.vi"("告警代码"=w413, "故障代码"=w414, "运行步序"=w418, "参数"=w416) -> ("报警内容"=w417:T19)  [unwired: 6 in, 1 out]
        n213 = And(x=w410, y=w409) -> (x .and. y?=w408:bool)
        n214 = case shown="真" w408 {
          tunnel: w417 -> [_ w428]
          tunnel: w415 -> [_ w427]
          frame False {
          }
          frame True {
            n215 = Unbundle By Name(w428) -> ("参数"=w423:string, "报警内容"=w422:string, "报警分析"=w421:string)
            n216 = Get Date/Time In Seconds() -> (seconds since 1Jan1904=w426:timestamp)
            n217 = Bundle("报警内容"=w422, "报警分析"=w421) -> (w420:cluster{"报警内容":string, "报警分析":string})  [unwired: 1 in]
            n218 = Bundle By Name(cluster=T18 {"时间标识"=timestamp(0 s since 1904-01-01), "设备"="", "日志信息"="", "备注"=""} ("data in"), "时间标识"=w426, "设备"=w423, "日志信息"=w422, "备注"=w421) -> (w425:T18)
            n219 = call "balloon入队列.vi"("报警内容"=w420, "队列"=w427) -> ()  [unwired: 9 in, 1 out]
            n220 = call "总磷总氮报警信息.vi"("data in"=w425) -> ()  [unwired: 10 in, 1 out]
          }
        }
      }
    }
  }
  n221 = Read from Text File(file (use dialog)=w4) -> (text=w5:string)  [unwired: 3 in, 3 out]
  n222 = while {
    shift-right: [w431] -> _
    shift-left: w5 -> [w433]
    tunnel: w4 -> [w430]
    stop <- FALSE stop-if-true
    n223 = Read from Text File(file (use dialog)=w430) -> (text=w431:string)  [unwired: 3 in, 3 out]
    n224 = Not Equal?(x=w433, y=w431) -> (x != y?=w432:bool)
    n225 = Wait (ms)(milliseconds to wait=u32 1000 ("等待时间（毫秒）")) -> ()  [unwired: 1 out]
    n226 = case shown="真" w432 {
      tunnel: w430 -> [_ w435]
      frame False {
      }
      frame True {
        n227 = vi-ref "总磷总氮断电保存全局变量.vi"() -> (w439:refnum<vi>)
        n228 = call <vilib>:"Open Config Data.vi"("configuration file path"=w435) -> ("error out"=w437:errorcluster, "refnum"=w440:T14)  [unwired: 8 in, 1 out]
        n229 = call <userlib>:"Read Panel from INI__ogtk.vi"("error in (no error)"=w437, "VI ref"=w439, "refnum"=w440) -> ("error out"=w436:errorcluster, "refnum out"=w438:T14)  [unwired: 7 in]
        n230 = call <vilib>:"Close Config Data.vi"("error in (no error)"=w436, "refnum"=w438) -> ()  [unwired: 8 in, 2 out]
      }
    }
  }
  n231 = while {
    tunnel: w11 -> [_]
    stop <- FALSE stop-if-true
    # "试剂填充 172 \n管路清洗108\n氨氮92\n总磷131\n总磷海水147\n总氮76\n总氮海水92"
    n232 = global read "VAR总磷总氮全局变量.vi" "状态告警区"() -> (w467:T7)
    n233 = global read "VAR总磷总氮全局变量.vi" "状态告警区"() -> (w465:T7)
    n234 = global read "VAR总磷总氮全局变量.vi" "状态告警区"() -> (w471:T7)
    n235 = global read "VAR总磷总氮全局变量.vi" "状态告警区"() -> (w463:T7)
    n236 = Wait (ms)(milliseconds to wait=u32 1000 ("等待时间（毫秒）")) -> ()  [unwired: 1 out]
    n237 = Unbundle By Name(w471) -> ("id"=w468:u16, "flowid"=w470:u16, "量程"=w469:u16, "工作状态"=w456:T9, "F0"=→"F0":sgl, "F1"=→"F1":sgl, "F2"=→"F2":sgl, "F3"=→"F3":sgl, "ADC"=→"ADC":sgl, "总磷控温温度1"=→"温度1":sgl, "营养盐控温温度2"=→"温度2":sgl)
    n238 = Unbundle By Name(w463) -> ("日志代码"=w462:u16)
    n239 = Unbundle By Name(w467) -> ("日志代码"=w459:u16)
    n240 = Unbundle By Name(w465) -> ("工作状态"=w451:T9, "id"=w452:u16)
    n241 = case shown="\"空闲\"" w451 {
      frame "空闲" {
        n242 = local write "数组"(string[] [] ("数组")) -> ()
      }
      frame "水样测试", Default {
      }
    }
    n243 = feedback-in #2(w459) -> ()
    n244 = feedback #2(w459) -> (w476:u16)
    n245 = feedback #3(w462) -> (w464:u16)
    n246 = feedback-in #3(w462) -> ()
    n247 = Not Equal To 0?(x=w451) -> (x != 0?=w449:bool)
    n248 = Subtract(x=w459, y=1) -> (x-y=→"多列列表框":i32)
    n249 = Not Equal?(x=w459, y=w476) -> (x != y?=w475:bool)
    n250 = call <vilib>:"Boolean Crossing PtByPt.vi"("direction"=enum16{"either", "false-true", "true-false"}."false-true", "input"=w449) -> ("crossing"=w453:bool)  [unwired: 1 in]
    n251 = call <vilib>:"Boolean Crossing PtByPt.vi"("direction"=enum16{"either", "false-true", "true-false"}."true-false", "input"=w449) -> ("crossing"=w448:bool)  [unwired: 1 in]
    n252 = Not Equal To 0?(x=w456) -> (x != 0?=w473:bool)
    n253 = case shown="假" w475 {
      tunnel: w459 -> [_ w612]
      frame False {
      }
      frame True {
        n254 = Subtract(x=w612, y=1) -> (x-y=w610:i32)
        n255 = Subtract(x=w610, y=5) -> (x-y=w614:i32)
        n256 = Greater Or Equal To 0?(x=w614) -> (x >= 0?=w613:bool)
        n257 = property on="多列列表框" class="MCListbox (严格)"() -> (error out=w618:errorcluster, "TopLeft"=w619:T22)  [unwired: 2 in, 1 out]
        n258 = Select(t=w614, s=w613, f=0) -> (s? t:f=w615:i32)
        n259 = Bundle By Name(cluster=w619, "Row"=w615) -> (w620:T22)
        n260 = property on="多列列表框" class="MCListbox (严格)"(error in=w618, "TopLeft"=w620) -> ()  [unwired: 1 in, 2 out]
      }
    }
    n261 = case shown="真" w453 {
      tunnel: w451 -> [_ w502]
      tunnel: w452 -> [_ w499]
      frame False {
      }
      frame True {
        n262 = case shown="\"空闲\", 默认" w502 {
          tunnel: [_ "【水样测试】" ("字符串") "【标样核查】" ("字符串") "【零点核查】" ("字符串") "【跨度核查】" ("字符串") "【空白测试】" ("字符串") "【平行样测试】" ("字符串") "【加标回收】" ("字符串") "【空白校准】" ("字符串") "【标样校准】" ("字符串")] -> w507
          frame "空闲", Default {
          }
          frame "水样测试" {
          }
          frame "标样核查" {
          }
          frame "零点核查" {
          }
          frame "跨度核查" {
          }
          frame "空白测试" {
          }
          frame "平行样测试" {
          }
          frame "加标回收" {
          }
          frame "空白校准" {
          }
          frame "标样校准" {
          }
        }
        n263 = call "id参数转换.vi"("id"=w499) -> ("table输出"=w498:string)  [unwired: 10 in]
        n264 = Concatenate Strings("-->>" ("字符串"), w507, "启动" ("字符串")) -> (w506:string)
        n265 = Get Date/Time In Seconds() -> (seconds since 1Jan1904=w504:timestamp)
        n266 = Bundle By Name(cluster=T21 {"时间标识"=timestamp(0 s since 1904-01-01), "设备"="", "日志信息"="", "流程参数"=""} ("data in"), "时间标识"=w504, "设备"=w498, "日志信息"=w506) -> (w503:T21)
        n267 = call "总磷总氮操作日志.vi"("data in"=w503) -> ()  [unwired: 11 in]
      }
    }
    n268 = case shown="真" w448 {
      tunnel: w451 -> [_ w483]
      tunnel: w452 -> [_ w480]
      frame False {
      }
      frame True {
        n269 = case shown="\"水样测试\"" w483 {
          tunnel: [_ "【水样测试】" ("字符串") "【标样核查】" ("字符串") "【零点核查】" ("字符串") "【跨度核查】" ("字符串") "【空白测试】" ("字符串") "【平行样测试】" ("字符串") "【加标回收】" ("字符串") "【空白校准】" ("字符串") "【标样校准】" ("字符串")] -> w488
          frame "空闲", Default {
          }
          frame "水样测试" {
          }
          frame "标样核查" {
          }
          frame "零点核查" {
          }
          frame "跨度核查" {
          }
          frame "空白测试" {
          }
          frame "平行样测试" {
          }
          frame "加标回收" {
          }
          frame "空白校准" {
          }
          frame "标样校准" {
          }
        }
        n270 = call "id参数转换.vi"("id"=w480) -> ("table输出"=w479:string)  [unwired: 10 in]
        n271 = Concatenate Strings("-->>" ("字符串"), w488, "停止" ("字符串")) -> (w487:string)
        n272 = Get Date/Time In Seconds() -> (seconds since 1Jan1904=w485:timestamp)
        n273 = Bundle By Name(cluster=T21 {"时间标识"=timestamp(0 s since 1904-01-01), "设备"="", "日志信息"="", "流程参数"=""} ("data in"), "时间标识"=w485, "设备"=w479, "日志信息"=w487) -> (w484:T21)
        n274 = call "总磷总氮操作日志.vi"("data in"=w484) -> ()  [unwired: 11 in]
      }
    }
    n275 = call <vilib>:"Boolean Crossing PtByPt.vi"("input"=w473) -> ("crossing"=w455:bool)  [unwired: 2 in]
    n276 = Bundle By Name(cluster=T20 {"启动模式"=enum."跨度核查", "启动参数"=1, "量程"=enum."低量程"} ("参数簇"), "启动参数"=w468, "启动模式"=w470, "量程"=w469) -> (w466:T20)
    n277 = First Call?() -> (First Call?: T/F=w474:bool)
    n278 = Or(x=w455, y=w474) -> (x .or. y?=w472:bool)
    n279 = while {
      tunnel: w472 -> [w598]
      tunnel: w466 -> [w597]
      shift-right: [w592] -> _
      shift-left: _ -> [w594]
      shift-right: [w593] -> _
      shift-left: _ -> [w595]
      shift-right: ["流程路径"] -> _
      shift-left: _ -> [w590]
      stop <- TRUE stop-if-true
      n280 = Not Equal?(x=w590, y="流程路径") -> (x != y?=w588:bool)
      n281 = Or(x=w598, y=w588) -> (x .or. y?=w589:bool)
      n282 = case shown="真" w589 {
        tunnel: [w600 w608] -> w593
        tunnel: [w599 w607] -> w592
        tunnel: w597 -> [_ w602]
        tunnel: w595 -> [w600 _]
        tunnel: w594 -> [w599 _]
        tunnel: "流程路径" -> [_ w601]
        frame False {
        }
        frame True {
          n283 = call "斯坦道XML解析.vi"("添加的路径"=w601, "参数簇"=w602) -> ("步骤时间"=w603:string[], "步骤名"=w605:string[])  [unwired: 8 in]
          n284 = Build Array(w605, w603) -> (w604:string[][])
          n285 = for {
            tunnel: w605 -> [_] mode=indexing
            tunnel: [w609] -> w606 mode=indexing
            i -> [w609]
          }
          n286 = Transpose 2D Array(2D array=w604) -> (transposed array=w607:string[][])
          n287 = Number To Decimal String(number=w606) -> (decimal integer string=w608:string[])  [unwired: 1 in]
        }
      }
      n288 = property on="多列列表框" class="MCListbox (严格)"("ItemNames"=w592, "RowHdrs[]"=w593) -> ()  [unwired: 2 in, 2 out]
    }
    n289 = Not Equal?(x=w462, y=w464) -> (x != y?=w461:bool)
    n290 = case shown="真" w461 {
      frame False {
      }
      frame True {
        n291 = property on="多列列表框" class="MCListbox (严格)"() -> ("ItemNames"=w522:string[][], "Value"=w518:i32)  [unwired: 2 in, 2 out]
        n292 = Index Array(array=w522, index (row)=w518) -> (element=w521:string[])  [unwired: 1 in]
        n293 = Index Array(array=w521) -> (element=w520:string)  [unwired: 1 in]
        n294 = call "过滤筛选流程.vi"("字符串"=w520) -> ("匹配后偏移量"=w519:i32)  [unwired: 10 in]
        n295 = case shown="默认" w519 {
          tunnel: w520 -> [w524 _]
          tunnel: w518 -> [w523 _]
          frame Default {
            n296 = case shown="默认" w524 {
              selector: w524 -> [w530 w537]
              tunnel: [w530 w537] -> w526
              tunnel: [string[] [] ("数组") w532] -> w525
              tunnel: w523 -> [_ w536]
              frame "读数" {
              }
              frame Default {
                n297 = Equal?(x=w536, y=1) -> (x = y?=w534:bool)
                n298 = Select(t=string[] [], s=w534, f="数组") -> (s? t:f=w532:string[])
              }
            }
            n299 = for {
              N: 1 -> [_]
              tunnel: w526 -> [w539]
              shift-right: [w538] -> w527
              shift-left: w525 -> [w540]
              n300 = Search 1D Array(1D array=w540, element=w539) -> (index of element=w543:i32)  [unwired: 1 in]
              n301 = Format Into String(format string="%s" ("格式字符串"), w539) -> (resulting string=w544:string)  [unwired: 2 in, 1 out]
              n302 = Equal?(x=w543, y=-1) -> (x = y?=w541:bool)
              n303 = case shown="真" w541 {
                tunnel: w544 -> [_ w554]
                tunnel: w540 -> [w546 w558]
                tunnel: w539 -> [_ w557]
                tunnel: [w546 w556] -> w538
                frame False {
                }
                frame True {
                  n304 = case shown="\"结束\"" w554 {
                    selector: w554 -> [w581 w584 w587]
                    tunnel: [w581 w583 w586] -> w553
                    frame Default {
                    }
                    frame "初始化" {
                      n305 = Concatenate Strings("-->>" ("字符串"), w584) -> (w583:string)
                    }
                    frame "结束" {
                      n306 = Concatenate Strings("-->>" ("字符串"), w587) -> (w586:string)
                    }
                  }
                  n307 = Insert Into Array(array=w558, new element=w557) -> (w556:string[])  [unwired: 1 in]
                  n308 = global read "VAR总磷总氮全局变量.vi" "状态告警区"() -> (w552:T7)
                  n309 = Unbundle By Name(w552) -> ("工作状态"=w551:T9)
                  n310 = case shown="\"水样测试\"" w551 {
                    tunnel: [_ "【水样测试】" ("字符串") "【标样核查】" ("字符串") "【零点核查】" ("字符串") "【跨度核查】" ("字符串") "【空白测试】" ("字符串") "【平行样测试】" ("字符串") "【加标回收】" ("字符串") "【空白校准】" ("字符串") "【标样校准】" ("字符串")] -> w549
                    frame "空闲", Default {
                    }
                    frame "水样测试" {
                    }
                    frame "标样核查" {
                    }
                    frame "零点核查" {
                    }
                    frame "跨度核查" {
                    }
                    frame "空白测试" {
                    }
                    frame "平行样测试" {
                    }
                    frame "加标回收" {
                    }
                    frame "空白校准" {
                    }
                    frame "标样校准" {
                    }
                  }
                  n311 = global read "VAR总磷总氮全局变量.vi" "状态告警区"() -> (w571:T7)
                  n312 = global read "VAR总磷总氮全局变量.vi" "状态告警区"() -> (w568:T7)
                  n313 = Unbundle By Name(w568) -> ("F0"=w565:sgl, "F1"=w564:sgl, "F2"=w563:sgl, "F3"=w562:sgl, "id"=w561:u16, "flowid"=w560:u16, "量程"=w559:u16)
                  n314 = Unbundle By Name(w571) -> ("id"=w548:u16)
                  n315 = call "id参数转换.vi"("id"=w548) -> ("table输出"=w547:string)  [unwired: 10 in]
                  n316 = Concatenate Strings(w549, w553) -> (w550:string)
                  n317 = Format Into String(format string="F0=%#f,F1=%#f,F2=%#f,F3=%#f,Flow=%d-%-d-%-d" ("格式字符串"), w565, w564, w563, w562, w561, w560, w559) -> (resulting string=w566:string)  [unwired: 2 in, 1 out]
                  n318 = Get Date/Time In Seconds() -> (seconds since 1Jan1904=w569:timestamp)
                  n319 = Bundle By Name(cluster=T21 {"时间标识"=timestamp(0 s since 1904-01-01), "设备"="", "日志信息"="", "流程参数"=""} ("data in"), "时间标识"=w569, "设备"=w547, "日志信息"=w550, "流程参数"=w566) -> (w570:T21)
                  n320 = call "总磷总氮操作日志.vi"("data in"=w570) -> ()  [unwired: 11 in]
                }
              }
            }
            n321 = local write "数组"(w527) -> ()
          }
          frame -1 {
          }
        }
      }
    }
  }
  n322 = call "设置模块队列名.vi"() -> ("Msg"=w2:string)  [unwired: 5 in]
  n323 = Obtain Queue(name (unnamed)=w6, element data type=cluster{"命令":string, "data":variant} {"命令"="", "data"=variant}) -> (queue out=w7:refnum<queue>)  [unwired: 3 in, 2 out]
  n324 = Obtain Notifier(name (unnamed)=w2, notification data type=FALSE) -> (notifier out=w1:refnum<notifier>)  [unwired: 2 in, 2 out]
  n325 = control-ref of="测量模式下拉列表"() -> (w14:refnum<vi>)
  n326 = while {
    tunnel: w7 -> [w625]
    tunnel: [w623] -> _
    stop <- FALSE stop-if-true
    # "定时更新"
    n327 = Get Queue Status(queue=w625) -> (queue out=w622:refnum<queue>, # elements in queue=w621:i32)  [unwired: 2 in, 6 out]
    n328 = Wait (ms)(milliseconds to wait=u32 1000 ("等待时间（毫秒）")) -> ()  [unwired: 1 out]
    n329 = case shown="0" w621 {
      tunnel: w622 -> [_ w633]
      tunnel: [_ w631] -> w623
      frame Default {
      }
      frame 0 {
        n330 = global read "VAR总磷总氮全局变量.vi" "启动队列名称"() -> (w629:cluster{"String":string, "Value":u16}[])
        n331 = Index Array(array=w629) -> (element=w628:cluster{"String":string, "Value":u16})  [unwired: 1 in]
        n332 = Unbundle By Name(w628) -> ("Value"=w627:u16)
        n333 = call "总磷总氮版本号读取.vi"("Slave ID"=w627) -> ("error out"=w631:errorcluster, "固件版本号"=→"固件版本号":string)  [unwired: 9 in]
        n334 = Bundle By Name(cluster=cluster{"命令":string, "data":variant} {"命令"="", "data"=variant} ("元素"), "命令"="读序列号", "data"=w627) -> (w632:cluster{"命令":string, "data":variant})
        n335 = Enqueue Element(queue=w633, element=w632) -> ()  [unwired: 2 in, 3 out]
      }
    }
  }
  n336 = while {
    tunnel: w7 -> [w641]
    stop <- FALSE stop-if-true
    n337 = Get Queue Status(queue=w641) -> (queue out=w639:refnum<queue>, # elements in queue=w638:i32)  [unwired: 2 in, 6 out]
    n338 = Wait (ms)(milliseconds to wait=u32 1000 ("等待时间（毫秒）")) -> ()  [unwired: 1 out]
    n339 = case shown="0" w638 {
      tunnel: w639 -> [_ w657]
      frame Default {
      }
      frame 0 {
        n340 = global read "VAR总磷总氮全局变量.vi" "启动队列名称"() -> (w646:cluster{"String":string, "Value":u16}[])
        n341 = for {
          tunnel: [w675] -> w647 mode=indexing
          tunnel: w646 -> [w676] mode=indexing
          n342 = Unbundle By Name(w676) -> ("Value"=w675:u16)
        }
        n343 = global read "VAR总磷总氮全局变量.vi" "状态告警区"() -> (w649:T7)
        n344 = Unbundle By Name(w649) -> ("系统时间"=w656:timestamp, "工作状态"=w648:T9)
        n345 = for {
          tunnel: w648 -> [w661]
          shift-right: [w662] -> w650
          shift-left: w657 -> [w664]
          tunnel: w647 -> [w658] mode=indexing
          n346 = Equal?(x=w661, y=T9."空闲") -> (x = y?=w659:bool)
          n347 = Bundle By Name(cluster=cluster{"命令":string, "data":variant} {"命令"="", "data"=variant} ("元素"), "命令"="读状态告警区", "data"=w658) -> (w666:cluster{"命令":string, "data":variant})
          n348 = Enqueue Element(queue=w664, element=w666) -> (queue out=w663:refnum<queue>)  [unwired: 2 in, 2 out]
          n349 = case shown="真" w659 {
            tunnel: w663 -> [w668 w671]
            tunnel: w658 -> [_ w670]
            tunnel: [w668 w669] -> w662
            frame False {
            }
            frame True {
              n350 = Bundle By Name(cluster=cluster{"命令":string, "data":variant} {"命令"="", "data"=variant} ("元素"), "命令"="读测量数据区", "data"=w670) -> (w673:cluster{"命令":string, "data":variant})
              n351 = Enqueue Element(queue=w671, element=w673) -> (queue out=w669:refnum<queue>)  [unwired: 2 in, 2 out]
            }
          }
        }
        n352 = Get Date/Time In Seconds() -> (seconds since 1Jan1904=w655:timestamp)
        n353 = Subtract(x=w655, y=w656) -> (x-y=w654:dbl)
        n354 = Absolute Value(x=w654) -> (abs(x)=w653:dbl)
        n355 = Greater Or Equal?(x=w653, y=120.0) -> (x >= y?=w651:bool)
        n356 = case shown="真" w651 {
          tunnel: w650 -> [_ w678]
          frame False {
          }
          frame True {
            n357 = call "总磷总氮启动命令.vi"("参数"=T23 {"站号"=3, "量程切换"=enum."AUTO", "控制命令"=enum."校时", "模式设置"=enum."待机", "测量间隔"=0}) -> ("启动命令"=w677:cluster{"命令":string, "data":variant})  [unwired: 10 in]
            n358 = Enqueue Element(queue=w678, element=w677) -> ()  [unwired: 2 in, 3 out]
          }
        }
      }
    }
    n359 = global read "总磷总氮断电保存全局变量.vi" "流程路径"() -> (w640:path)
    n360 = local write "流程路径"(w640) -> ()
    n361 = global read "总磷总氮断电保存全局变量.vi" "MB通信方式选择"() -> (w637:enum16{"串口", "TCP"})
    n362 = case shown="\"串口\", 默认" w637 {
      tunnel: [w644 w645] -> w636
      frame "串口", Default {
        n363 = global read "总磷总氮断电保存全局变量.vi" "VISA Resource"() -> (w644:refnum<visa-resource-name>)
      }
      frame "TCP" {
        n364 = global read "总磷总氮断电保存全局变量.vi" "IP"() -> (w645:string)
      }
    }
    "字符串 2" <- w636
  }
  n365 = control-ref of="量程参数读取"() -> (w12:refnum<vi>)
  n366 = control-ref of="参数下拉列表"() -> (w15:refnum<vi>)
  n367 = control-ref of="量程下拉列表"() -> (w16:refnum<vi>)
  n368 = control-ref of="公式"() -> (w13:refnum<vi>)
  n369 = while {
    tunnel: w7 -> [w686]
    tunnel: w16 -> [w685]
    tunnel: w15 -> [w684]
    tunnel: w14 -> [w683]
    tunnel: w13 -> [w682]
    tunnel: w12 -> [w681]
    tunnel: w1 -> [w680]
    stop <- FALSE stop-if-true
    n370 = event shown="[1] \"灯值调整\": 值改变" {
      selector: _ -> [_ _ _ _ _ _ _ _ _ _ _ _ _ _ _ _ _ _ _ _ _ _ _ _]
      dyn-events: _ -> [_ _ _ _ _ _ _ _ _ _ _ _ _ _ _ _ _ _ _ _ _ _ _ _]
      timeout: _ -> [_ _ _ _ _ _ _ _ _ _ _ _ _ _ _ _ _ _ _ _ _ _ _ _]
      tunnel: w686 -> [_ _ _ _ _ _ w706 w732 _ _ _ _ _ _ w829 _ w838 _ _ _ _ _ _ _]
      tunnel: w685 -> [_ _ _ _ _ _ _ _ _ w752 _ _ _ _ _ _ _ _ _ _ w854 _ _ _]
      tunnel: w684 -> [_ _ _ _ _ _ _ _ _ w756 _ _ _ w807 _ _ _ _ _ _ w852 _ w905 w912]
      tunnel: w683 -> [_ _ _ _ _ _ _ _ _ w754 _ _ _ _ _ _ _ _ _ _ w853 _ _ _]
      tunnel: w682 -> [_ _ _ _ _ _ _ _ _ _ _ _ _ _ _ _ _ _ _ _ w848 _ _ _]
      tunnel: w681 -> [_ _ _ _ _ _ _ _ _ _ _ _ _ _ _ _ _ _ _ _ _ _ w903 _]
      tunnel: [_ _ _ _ w692 _ _ _ _ _ _ _ _ _ _ _ _ _ _ _ _ _ _ _] -> _
      tunnel: w680 -> [_ _ _ _ _ _ _ _ _ _ _ _ _ _ _ _ w834 _ _ _ _ _ _ _]
      event Timeout {
        n371 = event-data() -> ()  [unwired: 1 in, 3 out]
      }
      event "灯值调整": Value Change {
        n372 = event-data() -> ()  [unwired: 1 in, 6 out]
        n373 = call "灯值调整对话框.vi"() -> ()  [unwired: 12 in]
      }
      event "启动参数设置": Value Change {
        n374 = event-data() -> ()  [unwired: 1 in, 6 out]
        n375 = call "启动参数设置.vi"() -> ()  [unwired: 12 in]
      }
      event "布尔": Mouse Down {
        n376 = event-data() -> ("CtlRef"=w689:refnum<vi>)  [unwired: 1 in, 5 out]
        n377 = property class="Bool (严格)"(reference=w689) -> ("Value"=w688:bool)  [unwired: 1 in, 2 out]
        n378 = case shown="真" w688 {
          frame False {
            n379 = call "密码键盘.vi"() -> ("NewNumber"=→"输入密码":dbl)  [unwired: 1 in]
          }
          frame True {
            n380 = local write "输入密码"(u32 0 ("输入密码")) -> ()
          }
        }
      }
      event "测量模式下拉列表", "量程下拉列表", "参数下拉列表": Value Change {
        n381 = event-data() -> ()  [unwired: 1 in, 6 out]
        n382 = local read "测量模式下拉列表"() -> (w695:enum16{"水样测量", "零点核查", "跨度核查", "标样核查", "加标回收"})
        n383 = local read "参数下拉列表"() -> (w694:enum16{"COD", "氨氮", "总氮", "总磷"})
        n384 = local read "量程下拉列表"() -> (w696:enum16{"低量程", "高量程"})
        n385 = Bundle("参数下拉列表"=w694, "测量模式下拉列表"=w695, "量程下拉列表"=w696) -> (w693:T13)  [unwired: 1 in]
        n386 = property on="曲线模型" class="曲线模型 (严格)"("属性"=w693) -> (error out=w692:errorcluster)  [unwired: 2 in, 1 out]
      }
      event "流程固件": Value Change {
        n387 = event-data() -> ()  [unwired: 1 in, 6 out]
        n388 = call "流程固件设置对话框.vi"() -> ()  [unwired: 12 in]
      }
      event "串口设置": Value Change {
        n389 = event-data() -> ()  [unwired: 1 in, 6 out]
        n390 = global read "总磷总氮断电保存全局变量.vi" "MB通信方式选择"() -> (w697:enum16{"串口", "TCP"})
        n391 = global read "总磷总氮断电保存全局变量.vi" "VISA Resource"() -> (w703:refnum<visa-resource-name>)
        n392 = global read "总磷总氮断电保存全局变量.vi" "PORT"() -> (w701:string)
        n393 = global read "总磷总氮断电保存全局变量.vi" "IP"() -> (w702:string)
        n394 = call "串口配置.vi"("PORT"=w701, "IP"=w702, "MB通信方式选择"=w697, "请选择串口:"=w703) -> ("PORT 2"=w699:string, "IP 2"=w700:string, "确认 2"=w704:bool, "VISA资源名称 2"=w705:refnum<visa-resource-name>, "MB通信方式选择 2"=w698:enum16{"串口", "TCP"})  [unwired: 3 in]
        n395 = case shown="真" w704 {
          tunnel: w705 -> [_ w711]
          tunnel: w706 -> [_ w710]
          tunnel: w700 -> [_ w709]
          tunnel: w699 -> [_ w708]
          tunnel: w698 -> [_ w707]
          frame False {
          }
          frame True {
            n396 = flat-sequence {
              tunnel: w711 -> [w716]
              tunnel: w710 -> [w717]
              tunnel: w709 -> [w715]
              tunnel: w708 -> [w714]
              tunnel: w707 -> [w713]
              frame #0 {
                n397 = global write "总磷总氮断电保存全局变量.vi" "IP"(w715) -> ()
                n398 = global write "总磷总氮断电保存全局变量.vi" "PORT"(w714) -> ()
                n399 = global write "总磷总氮断电保存全局变量.vi" "VISA Resource"(w716) -> ()
                n400 = global write "总磷总氮断电保存全局变量.vi" "MB通信方式选择"(w713) -> ()
                n401 = Flush Queue(queue=w717) -> (queue out=w712:refnum<queue>)  [unwired: 1 in, 2 out]
                n402 = Enqueue Element(queue=w712, element=cluster{"命令":string, "data":variant} {"命令"="启用模块", "data"=variant} ("元素")) -> ()  [unwired: 2 in, 3 out]
              }
              frame #1 {
                n403 = call "配置文件路径.vi"() -> ("appended path"=w719:path)  [unwired: 11 in]
                n404 = call <vilib>:"Open Config Data.vi"("configuration file path"=w719) -> ("error out"=w727:errorcluster, "refnum"=w730:T14)  [unwired: 8 in, 1 out]
                n405 = vi-ref "总磷总氮断电保存全局变量.vi"() -> (w729:refnum<vi>)
                n406 = call <userlib>:"Write Panel to INI__ogtk.vi"("error in (no error)"=w727, "VI ref"=w729, "refnum"=w730) -> ("error out"=w726:errorcluster, "refnum out"=w728:T14)  [unwired: 7 in]
                n407 = call <vilib>:"Close Config Data.vi"("error in (no error)"=w726, "refnum"=w728) -> ("error out"=w721:errorcluster, "file path"=w720:path)  [unwired: 8 in]
                n408 = Open/Create/Replace File(file path (use dialog)=w720, error in=w721) -> (refnum out=w724:refnum<file>, error out=w725:errorcluster)  [unwired: 4 in, 1 out]
                n409 = Flush File(refnum=w724, error in=w725) -> (refnum out=w723:refnum<file>, error out=w722:errorcluster)
                n410 = Close File(refnum=w723, error in=w722) -> ()  [unwired: 2 out]
              }
            }
          }
        }
      }
      event "模块启用": Value Change {
        n411 = event-data() -> ("OldVal"=w733:bool)  [unwired: 1 in, 5 out]
        n412 = Flush Queue(queue=w732) -> (queue out=w731:refnum<queue>)  [unwired: 1 in, 2 out]
        n413 = case shown="假" w733 {
          tunnel: w731 -> [w734 w736]
          frame False {
            n414 = Enqueue Element(queue=w734, element=cluster{"命令":string, "data":variant} {"命令"="停用模块", "data"=variant} ("元素")) -> ()  [unwired: 2 in, 3 out]
          }
          frame True {
            n415 = Enqueue Element(queue=w736, element=cluster{"命令":string, "data":variant} {"命令"="启用模块", "data"=variant} ("元素")) -> ()  [unwired: 2 in, 3 out]
          }
        }
      }
      event "流程路径": Value Change {
        n416 = event-data() -> ()  [unwired: 1 in, 6 out]
        n417 = flat-sequence {
          frame #0 {
            n418 = local read "流程路径"() -> (w738:path)
            n419 = global write "总磷总氮断电保存全局变量.vi" "流程路径"(w738) -> ()
          }
          frame #1 {
            n420 = call "配置文件路径.vi"() -> ("appended path"=w739:path)  [unwired: 11 in]
            n421 = call <vilib>:"Open Config Data.vi"("configuration file path"=w739) -> ("error out"=w747:errorcluster, "refnum"=w750:T14)  [unwired: 8 in, 1 out]
            n422 = vi-ref "总磷总氮断电保存全局变量.vi"() -> (w749:refnum<vi>)
            n423 = call <userlib>:"Write Panel to INI__ogtk.vi"("error in (no error)"=w747, "VI ref"=w749, "refnum"=w750) -> ("error out"=w746:errorcluster, "refnum out"=w748:T14)  [unwired: 7 in]
            n424 = call <vilib>:"Close Config Data.vi"("error in (no error)"=w746, "refnum"=w748) -> ("error out"=w741:errorcluster, "file path"=w740:path)  [unwired: 8 in]
            n425 = Open/Create/Replace File(file path (use dialog)=w740, error in=w741) -> (refnum out=w744:refnum<file>, error out=w745:errorcluster)  [unwired: 4 in, 1 out]
            n426 = Flush File(refnum=w744, error in=w745) -> (refnum out=w743:refnum<file>, error out=w742:errorcluster)
            n427 = Close File(refnum=w743, error in=w742) -> ()  [unwired: 2 out]
          }
        }
      }
      event "公式一键写入": Value Change {
        n428 = event-data() -> ()  [unwired: 1 in, 6 out]
        n429 = property class="Enum (严格)"(reference=w756) -> ("Value"=w755:enum16{"COD", "氨氮", "总氮", "总磷"})  [unwired: 1 in, 2 out]
        n430 = property class="Enum (严格)"(reference=w754) -> ("Value"=w753:enum16{"水样测量", "零点核查", "跨度核查", "标样核查", "加标回收"})  [unwired: 1 in, 2 out]
        n431 = property class="Enum (严格)"(reference=w752) -> ("Value"=w751:enum16{"低量程", "高量程"})  [unwired: 1 in, 2 out]
        n432 = local read "公式"() -> (w758:cluster{"X^2":dbl, "X":dbl, "b":dbl})
        n433 = call "公式复合写入.vi"("公式"=w758, "量程下拉列表"=w751, "测量模式下拉列表"=w753, "参数下拉列表"=w755) -> ("模型复制"=w757:T24)  [unwired: 7 in]
        n434 = invoke on="曲线模型" class="曲线模型 (严格)" method="模型复制.vi"("模型复制"=w757) -> ()  [unwired: 3 in, 4 out]
      }
      event "曲线模型": Value Change {
        n435 = event-data() -> ()  [unwired: 1 in, 6 out]
        n436 = Unbundle By Name("曲线模型") -> ("X^2"=w762:dbl, "X"=w761:dbl, "B"=w760:dbl)
        n437 = Bundle("X^2"=w762, "X"=w761, "B"=w760) -> (w759:cluster{"X^2":dbl, "X":dbl, "B":dbl})  [unwired: 1 in]
        n438 = local write "公式"(w759) -> ()
      }
      event "质控参数设置": Value Change {
        n439 = event-data() -> ()  [unwired: 1 in, 6 out]
        n440 = global read "总磷总氮断电保存全局变量.vi" "质控参数设置"() -> (w766:T25)
        n441 = call "总磷总氮质控参数设置.vi"("质控参数设置"=w766) -> ("质控参数设置 2"=w764:T25, "check？"=w765:bool)  [unwired: 9 in]
        n442 = case shown="真" w765 {
          tunnel: w766 -> [_ w768]
          tunnel: w764 -> [_ w767]
          frame False {
          }
          frame True {
            n443 = flat-sequence {
              tunnel: w768 -> [_]
              tunnel: w767 -> [w769]
              frame #0 {
                n444 = global write "总磷总氮断电保存全局变量.vi" "质控参数设置"(w769) -> ()
              }
              frame #1 {
                n445 = call "配置文件路径.vi"() -> ("appended path"=w770:path)  [unwired: 11 in]
                n446 = call <vilib>:"Open Config Data.vi"("configuration file path"=w770) -> ("error out"=w778:errorcluster, "refnum"=w781:T14)  [unwired: 8 in, 1 out]
                n447 = vi-ref "总磷总氮断电保存全局变量.vi"() -> (w780:refnum<vi>)
                n448 = call <userlib>:"Write Panel to INI__ogtk.vi"("error in (no error)"=w778, "VI ref"=w780, "refnum"=w781) -> ("error out"=w777:errorcluster, "refnum out"=w779:T14)  [unwired: 7 in]
                n449 = call <vilib>:"Close Config Data.vi"("error in (no error)"=w777, "refnum"=w779) -> ("error out"=w772:errorcluster, "file path"=w771:path)  [unwired: 8 in]
                n450 = Open/Create/Replace File(file path (use dialog)=w771, error in=w772) -> (refnum out=w775:refnum<file>, error out=w776:errorcluster)  [unwired: 4 in, 1 out]
                n451 = Flush File(refnum=w775, error in=w776) -> (refnum out=w774:refnum<file>, error out=w773:errorcluster)
                n452 = Close File(refnum=w774, error in=w773) -> ()  [unwired: 2 out]
              }
            }
          }
        }
      }
      event "仪器参数": Value Change {
        n453 = event-data() -> ()  [unwired: 1 in, 6 out]
        n454 = global read "总磷总氮断电保存全局变量.vi" "COD仪器参数"() -> (w787:T26)
        n455 = global read "总磷总氮断电保存全局变量.vi" "氨氮仪器参数"() -> (w786:T26)
        n456 = global read "总磷总氮断电保存全局变量.vi" "总氮仪器参数"() -> (w785:T26)
        n457 = global read "总磷总氮断电保存全局变量.vi" "总磷仪器参数"() -> (w784:T26)
        n458 = Bundle("COD仪器参数"=w787, "氨氮仪器参数"=w786, "总氮仪器参数"=w785, "总磷仪器参数"=w784) -> (w783:T27)  [unwired: 1 in]
        n459 = call "仪器参数设置.vi"("仪器参数"=w783) -> ("仪器参数 2"=w782:T27, "check？"=w788:bool)  [unwired: 9 in]
        n460 = case shown="真" w788 {
          tunnel: w782 -> [_ w789]
          frame False {
          }
          frame True {
            n461 = flat-sequence {
              tunnel: w789 -> [w794]
              frame #0 {
                n462 = Unbundle By Name(w794) -> ("COD仪器参数"=w792:T26, "氨氮仪器参数"=w791:T26, "总氮仪器参数"=w793:T26, "总磷仪器参数"=w790:T26)
                n463 = global write "总磷总氮断电保存全局变量.vi" "COD仪器参数"(w792) -> ()
                n464 = global write "总磷总氮断电保存全局变量.vi" "氨氮仪器参数"(w791) -> ()
                n465 = global write "总磷总氮断电保存全局变量.vi" "总氮仪器参数"(w793) -> ()
                n466 = global write "总磷总氮断电保存全局变量.vi" "总磷仪器参数"(w790) -> ()
              }
              frame #1 {
                n467 = call "配置文件路径.vi"() -> ("appended path"=w795:path)  [unwired: 11 in]
                n468 = call <vilib>:"Open Config Data.vi"("configuration file path"=w795) -> ("error out"=w803:errorcluster, "refnum"=w806:T14)  [unwired: 8 in, 1 out]
                n469 = vi-ref "总磷总氮断电保存全局变量.vi"() -> (w805:refnum<vi>)
                n470 = call <userlib>:"Write Panel to INI__ogtk.vi"("error in (no error)"=w803, "VI ref"=w805, "refnum"=w806) -> ("error out"=w802:errorcluster, "refnum out"=w804:T14)  [unwired: 7 in]
                n471 = call <vilib>:"Close Config Data.vi"("error in (no error)"=w802, "refnum"=w804) -> ("error out"=w797:errorcluster, "file path"=w796:path)  [unwired: 8 in]
                n472 = Open/Create/Replace File(file path (use dialog)=w796, error in=w797) -> (refnum out=w800:refnum<file>, error out=w801:errorcluster)  [unwired: 4 in, 1 out]
                n473 = Flush File(refnum=w800, error in=w801) -> (refnum out=w799:refnum<file>, error out=w798:errorcluster)
                n474 = Close File(refnum=w799, error in=w798) -> ()  [unwired: 2 out]
              }
            }
          }
        }
      }
      event "测试量程配置": Value Change {
        n475 = event-data() -> ()  [unwired: 1 in, 6 out]
        n476 = flat-sequence {
          tunnel: w807 -> [w810]
          frame #0 {
            n477 = property class="Enum (严格)"(reference=w810) -> ("Value"=w809:enum16{"COD", "氨氮", "总氮", "总磷"})  [unwired: 1 in, 2 out]
            n478 = case shown="默认" w809 {
              tunnel: "测试量程配置" -> [_ w811 w812 w813 w814]
              frame Default {
              }
              frame "COD" {
                n479 = global write "总磷总氮断电保存全局变量.vi" "COD自动测试量程配置"(w811) -> ()
              }
              frame "氨氮" {
                n480 = global write "总磷总氮断电保存全局变量.vi" "氨氮自动测试量程配置"(w812) -> ()
              }
              frame "总氮" {
                n481 = global write "总磷总氮断电保存全局变量.vi" "总氮自动测试量程配置"(w813) -> ()
              }
              frame "总磷" {
                n482 = global write "总磷总氮断电保存全局变量.vi" "总磷自动测试量程配置"(w814) -> ()
              }
            }
          }
          frame #1 {
            n483 = call "配置文件路径.vi"() -> ("appended path"=w815:path)  [unwired: 11 in]
            n484 = call <vilib>:"Open Config Data.vi"("configuration file path"=w815) -> ("error out"=w823:errorcluster, "refnum"=w826:T14)  [unwired: 8 in, 1 out]
            n485 = vi-ref "总磷总氮断电保存全局变量.vi"() -> (w825:refnum<vi>)
            n486 = call <userlib>:"Write Panel to INI__ogtk.vi"("error in (no error)"=w823, "VI ref"=w825, "refnum"=w826) -> ("error out"=w822:errorcluster, "refnum out"=w824:T14)  [unwired: 7 in]
            n487 = call <vilib>:"Close Config Data.vi"("error in (no error)"=w822, "refnum"=w824) -> ("error out"=w817:errorcluster, "file path"=w816:path)  [unwired: 8 in]
            n488 = Open/Create/Replace File(file path (use dialog)=w816, error in=w817) -> (refnum out=w820:refnum<file>, error out=w821:errorcluster)  [unwired: 4 in, 1 out]
            n489 = Flush File(refnum=w820, error in=w821) -> (refnum out=w819:refnum<file>, error out=w818:errorcluster)
            n490 = Close File(refnum=w819, error in=w818) -> ()  [unwired: 2 out]
          }
        }
      }
      event "手动启动": Value Change {
        n491 = event-data() -> ()  [unwired: 1 in, 6 out]
        n492 = call "总磷总氮启动参数对话框.vi"() -> ("确认"=w827:bool, "元素"=w828:cluster{"命令":string, "data":variant})  [unwired: 10 in]
        n493 = case shown="真" w827 {
          tunnel: w829 -> [_ w832]
          tunnel: w828 -> [_ w831]
          frame False {
          }
          frame True {
            n494 = Flush Queue(queue=w832) -> (queue out=w830:refnum<queue>)  [unwired: 1 in, 2 out]
            n495 = Enqueue Element(queue=w830, element=w831) -> ()  [unwired: 2 in, 3 out]
          }
        }
      }
      event "单步测试": Value Change {
        n496 = event-data() -> ()  [unwired: 1 in, 6 out]
        n497 = call "总磷单步调试对话框.vi"() -> ()  [unwired: 12 in]
      }
      event "停止": Value Change {
        n498 = event-data() -> ()  [unwired: 1 in, 6 out]
        n499 = Send Notification(notification=TRUE ("通知"), notifier=w834) -> ()  [unwired: 1 in, 2 out]
        n500 = Enqueue Element(queue=w838, element=cluster{"命令":string, "data":variant} {"命令"="启动", "data"=variant(cluster{"站号":u16, "控制命令输出":u16[]} {"站号"=1, "控制命令输出"=[2816]})} ("元素")) -> (queue out=w835:refnum<queue>)  [unwired: 2 in, 2 out]
        n501 = Enqueue Element(queue=w835, element=cluster{"命令":string, "data":variant} {"命令"="启动", "data"=variant(cluster{"站号":u16, "控制命令输出":u16[]} {"站号"=2, "控制命令输出"=[2816]})} ("元素")) -> ()  [unwired: 2 in, 3 out]
      }
      event "参数设置": Value Change {
        n502 = event-data() -> ()  [unwired: 1 in, 6 out]
        n503 = property on="窗格" class="Pane"("Origin"=T16 {"Horizontal"=0, "Vertical"=628} ("原点")) -> ()  [unwired: 2 in, 2 out]
      }
      event "返回": Value Change {
        n504 = event-data() -> ()  [unwired: 1 in, 6 out]
        n505 = property on="窗格" class="Pane"("Origin"=T16 {"Horizontal"=0, "Vertical"=0} ("原点")) -> ()  [unwired: 2 in, 2 out]
      }
      event "公式.X^2", "公式.X", "公式.b", "量程参数读取.测量精度", "量程参数读取.检出限", "量程参数读取.上限", "量程参数读取.下限", "量程参数读取.阈值（低->高）", "量程参数读取.阈值（高->低）", "量程参数读取.稀释度": Mouse Down {
        n506 = event-data() -> ("CtlRef"=w844:refnum<vi>)  [unwired: 1 in, 7 out]
        n507 = property class="DigNum (严格)"(reference=w844) -> (reference out=w842:refnum<vi>, "Value"=w843:dbl)  [unwired: 1 in, 1 out]
        n508 = call "数字键盘.vi"("OldNumber"=w843) -> ("NewNumber"=w841:dbl)
        n509 = property class="DigNum (严格)"(reference=w842, "Val(Sgnl)"=w841) -> ()  [unwired: 1 in, 2 out]
      }
      event "读公式": Value Change {
        n510 = event-data() -> ()  [unwired: 1 in, 6 out]
        n511 = property class="Enum (严格)"(reference=w852) -> ("Value"=w851:enum16{"COD", "氨氮", "总氮", "总磷"})  [unwired: 1 in, 2 out]
        n512 = property class="Enum (严格)"(reference=w853) -> ("Value"=w850:enum16{"水样测量", "零点核查", "跨度核查", "标样核查", "加标回收"})  [unwired: 1 in, 2 out]
        n513 = property class="Enum (严格)"(reference=w854) -> ("Value"=w849:enum16{"低量程", "高量程"})  [unwired: 1 in, 2 out]
        n514 = call "总磷总氮公式读取.vi"("量程"=w849, "测量模式"=w850, "测量参数"=w851) -> ("error out"=w846:errorcluster, "公式"=w847:cluster{"X^2":dbl, "X":dbl, "b":dbl})  [unwired: 7 in]
        n515 = property class="Clust (严格)"(reference=w848, "Value"=w847) -> ()  [unwired: 1 in, 2 out]
        n516 = case shown="错误" w846 {
          tunnel: ["读取成功" ("消息") "读取失败" ("消息")] -> w845
          frame No Error {
          }
          frame Error {
          }
        }
        n517 = One Button Dialog(message=w845) -> ()  [unwired: 1 in, 1 out]
      }
      event "写公式": Value Change {
        n518 = event-data() -> ()  [unwired: 1 in, 6 out]
        n519 = call "总磷总氮公式写入.vi"("公式"="公式", "量程"="量程下拉列表", "测量模式"="测量模式下拉列表", "测量参数"="参数下拉列表") -> ("error out"=w861:errorcluster)  [unwired: 7 in]
        n520 = case shown="无错误" w861 {
          tunnel: ["写入成功" ("消息") "写入失败" ("消息")] -> w862
          tunnel: "测量模式下拉列表" -> [w871 _]
          tunnel: "量程下拉列表" -> [w869 _]
          tunnel: "参数下拉列表" -> [w864 _]
          tunnel: "公式" -> [w863 _]
          frame No Error {
            n521 = Equal?(x=w871, y=enum16{"水样测量", "零点核查", "跨度核查", "标样核查", "加标回收"}."水样测量" ("测量模式下拉列表")) -> (x = y?=w867:bool)
            n522 = Equal?(x=w869, y=enum16{"低量程", "高量程"}."低量程" ("量程下拉列表")) -> (x = y?=w866:bool)
            n523 = And(x=w867, y=w866) -> (x .and. y?=w865:bool)
            n524 = case shown="真" w865 {
              tunnel: w864 -> [_ w874]
              tunnel: w863 -> [_ w873]
              frame False {
              }
              frame True {
                n525 = case shown="\"COD\"" w874 {
                  tunnel: w873 -> [w875 w881 w887 w893]
                  frame "总磷", Default {
                    n526 = Unbundle By Name(w875) -> ("X^2"=w878:dbl, "X"=w877:dbl, "b"=w876:dbl)
                    n527 = global read "总磷总氮断电保存全局变量.vi" "总磷仪器参数"() -> (w879:T26)
                    n528 = Bundle By Name(cluster=w879, "曲线截距"=w876, "曲线斜率"=w877, "二次多项式系数"=w878) -> (w880:T26)
                    n529 = global write "总磷总氮断电保存全局变量.vi" "总磷仪器参数"(w880) -> ()
                  }
                  frame "总氮" {
                    n530 = Unbundle By Name(w881) -> ("X^2"=w884:dbl, "X"=w883:dbl, "b"=w882:dbl)
                    n531 = global read "总磷总氮断电保存全局变量.vi" "总氮仪器参数"() -> (w885:T26)
                    n532 = Bundle By Name(cluster=w885, "曲线截距"=w882, "曲线斜率"=w883, "二次多项式系数"=w884) -> (w886:T26)
                    n533 = global write "总磷总氮断电保存全局变量.vi" "总氮仪器参数"(w886) -> ()
                  }
                  frame "COD" {
                    n534 = Unbundle By Name(w887) -> ("X^2"=w890:dbl, "X"=w889:dbl, "b"=w888:dbl)
                    n535 = global read "总磷总氮断电保存全局变量.vi" "COD仪器参数"() -> (w891:T26)
                    n536 = Bundle By Name(cluster=w891, "曲线截距"=w888, "曲线斜率"=w889, "二次多项式系数"=w890) -> (w892:T26)
                    n537 = global write "总磷总氮断电保存全局变量.vi" "COD仪器参数"(w892) -> ()
                  }
                  frame "氨氮" {
                    n538 = Unbundle By Name(w893) -> ("X^2"=w896:dbl, "X"=w895:dbl, "b"=w894:dbl)
                    n539 = global read "总磷总氮断电保存全局变量.vi" "氨氮仪器参数"() -> (w897:T26)
                    n540 = Bundle By Name(cluster=w897, "曲线截距"=w894, "曲线斜率"=w895, "二次多项式系数"=w896) -> (w898:T26)
                    n541 = global write "总磷总氮断电保存全局变量.vi" "氨氮仪器参数"(w898) -> ()
                  }
                }
              }
            }
          }
          frame Error {
          }
        }
        n542 = One Button Dialog(message=w862) -> ()  [unwired: 1 in, 1 out]
      }
      event "量程切换阈值读取": Value Change {
        n543 = event-data() -> ()  [unwired: 1 in, 6 out]
        n544 = property class="Enum (严格)"(reference=w905) -> ("Value"=w904:enum16{"COD", "氨氮", "总氮", "总磷"})  [unwired: 1 in, 2 out]
        n545 = call "总磷总氮量程读取.vi"("测量参数"=w904) -> ("error out"=w901:errorcluster, "量程参数读取"=w900:T28)  [unwired: 9 in]
        n546 = property class="Clust (严格)"(reference=w903, "Value"=w900) -> ()  [unwired: 1 in, 2 out]
        n547 = case shown="错误" w901 {
          tunnel: ["读取成功" ("消息") "读取失败" ("消息")] -> w902
          frame No Error {
          }
          frame Error {
          }
        }
        n548 = One Button Dialog(message=w902) -> ()  [unwired: 1 in, 1 out]
      }
      event "量程切换阈值写入": Value Change {
        n549 = event-data() -> ()  [unwired: 1 in, 6 out]
        n550 = property class="Enum (严格)"(reference=w912) -> ("Value"=w908:enum16{"COD", "氨氮", "总氮", "总磷"})  [unwired: 1 in, 2 out]
        n551 = call "总磷总氮量程写入.vi"("量程参数写入"="量程参数读取", "测量参数"=w908) -> ("error out"=w910:errorcluster)  [unwired: 8 in]
        n552 = case shown="无错误" w910 {
          tunnel: ["写入成功" ("消息") "写入失败" ("消息")] -> w911
          frame No Error {
          }
          frame Error {
          }
        }
        n553 = One Button Dialog(message=w911) -> ()  [unwired: 1 in, 1 out]
      }
    }
  }
